vi "CL-3000 sample.vi"() -> ()   [LabVIEW 2020]
uses:
  ctrl/select_out.ctl
  ctrl/select_group.ctl
  Public/enums/CL3IF_PEAKNO.ctl
  Public/clusters/CL3IF_ETHERNET_SETTING.ctl
  Public/enums/CL3IF_SELECTED_INDEX.ctl
  Public/enums/CL3IF_OUTNO.ctl
  Public/enums/CL3IF_ZERO_GROUP.ctl
  Keyence CL-3000.lvlib
panel:
  out "pulase_reset":bool=TRUE
  out "mask_left_1":bool
  in  "display point num":u16=2 min=2 max=10000
  out "data num":u16
  out "mask_right":bool
  out "No Wave":string="\nNo Wave"
  out "log1":dbl[][](graph)
  out "log2":dbl[][](graph)
  out "log3":dbl[][](graph)
  out "log4":dbl[][](graph)
  out "log5":dbl[][](graph)
  out "log6":dbl[][](graph)
  out "log7":dbl[][](graph)
  out "select_out_last":T1
  out "log8":dbl[][](graph)
  in  "timeout":u32=5000 caption="Timeout"
  in  "path":path
  out "mask_left_2":bool
  in  "on_off_group":bool
  out "Result_8":string caption="Result"
  out "Result_4":string caption="Result"
  out "Result_7":string caption="Result"
  in  "select_group":T2
  out "Result_5":string caption="Result"
  out "Result_6":string caption="Result"
  in  "light_ctrl_off":bool
  in  "light_ctrl_on":bool
  in  "meas_ctrl_off":bool
  in  "meas_ctrl_on":bool
  out "Result_2":string caption="Result"
  in  "peak4":bool
  in  "peak3":bool
  in  "peak2":bool
  in  "peak1":bool
  out "Light Graph":dbl[][](graph)
  in  "selectedIndex":enum16{"OLDEST", "NEWEST"}(ring)
  in  "request_data":u32=10000 caption="Request\nData" min=1 max=10000
  in  "save_csv_file":bool
  in  "select_out_graph":T1
  in  "select_out_command":T1
  in  "on_off":bool
  in  "reset_pulse_count":bool
  out "pulse_count":i32 caption="Pulse Count"
  in  "get_pulse_count":bool
  out "program_no":u8 caption="Get Program No"
  in  "get_program_no":bool
  in  "switch_program_no":u8 caption="Switch Program No" max=7
  in  "switch_program":bool
  out "Result_3":string caption="Result"
  in  "reset_group":bool
  in  "reset_multi":bool
  in  "timing_group":bool
  in  "timing_multi":bool
  in  "auto_zero_group":bool
  in  "auto_zero_multi":bool
  out "Result_1":string caption="Result"
  in  "IP Address":u8[](array[numeric])=[192, 168, 1, 1]
  in  "Comm Interface":enum8{"USB", "ETHERNET"}(ring)
  in  "LabVIEW stop":bool
  in  "clear_storage_data":bool
  in  "stop_storage":bool
  in  "start_storage":bool
  out "storage_index":u32 caption="Index"
  out "Measurement Data":T3(array[cluster])=[{"Out No"=1, "Value"=0, "valueInfo"=enum."VALID", "judgeResult"=0}, {"Out No"=2, "Value"=0, "valueInfo"=enum."VALID", "judgeResult"=0}, {"Out No"=3, "Value"=0, "valueInfo"=enum."VALID", "judgeResult"=0}, {"Out No"=4, "Value"=0, "valueInfo"=enum."VALID", "judgeResult"=0}, {"Out No"=5, "Value"=0, "valueInfo"=enum."VALID", "judgeResult"=0}, {"Out No"=6, "Value"=0, "valueInfo"=enum."VALID", "judgeResult"=0}, {"Out No"=7, "Value"=0, "valueInfo"=enum."VALID", "judgeResult"=0}, {"Out No"=8, "Value"=0, "valueInfo"=enum."VALID", "judgeResult"=0}] {"judgeResult" items=["HI"=1, "GO"=2, "LO"=4, "**"=5, "--"=0]}
  in  "get_light_stop":bool
  in  "get_trend_stop":bool
  in  "close":bool
  in  "Port":u32
  in  "Head":u8 max=5
  in  "get_light_start":bool
  in  "select_graph":enum8{"TriggerCount", "PulseCount"}(ring)
  in  "get_storage_data":bool
  in  "get_storage_index":bool
  in  "get_trend_start":bool
  out "trend_index":u32 caption="Index"
  in  "get_trend_index":bool
  in  "open":bool
  in  "Device ID":i32 min=0 max=2
  out "Trend Graph":T4(graph)
  # "Judgement\nResult"
  # "Measurement Data"
  # "ValueInfo"
  # "Out No"
  # "Value"
  # "ver 1.0.0"
  # "Trend DATA"
  # "Storage DATA"
  # "Light"
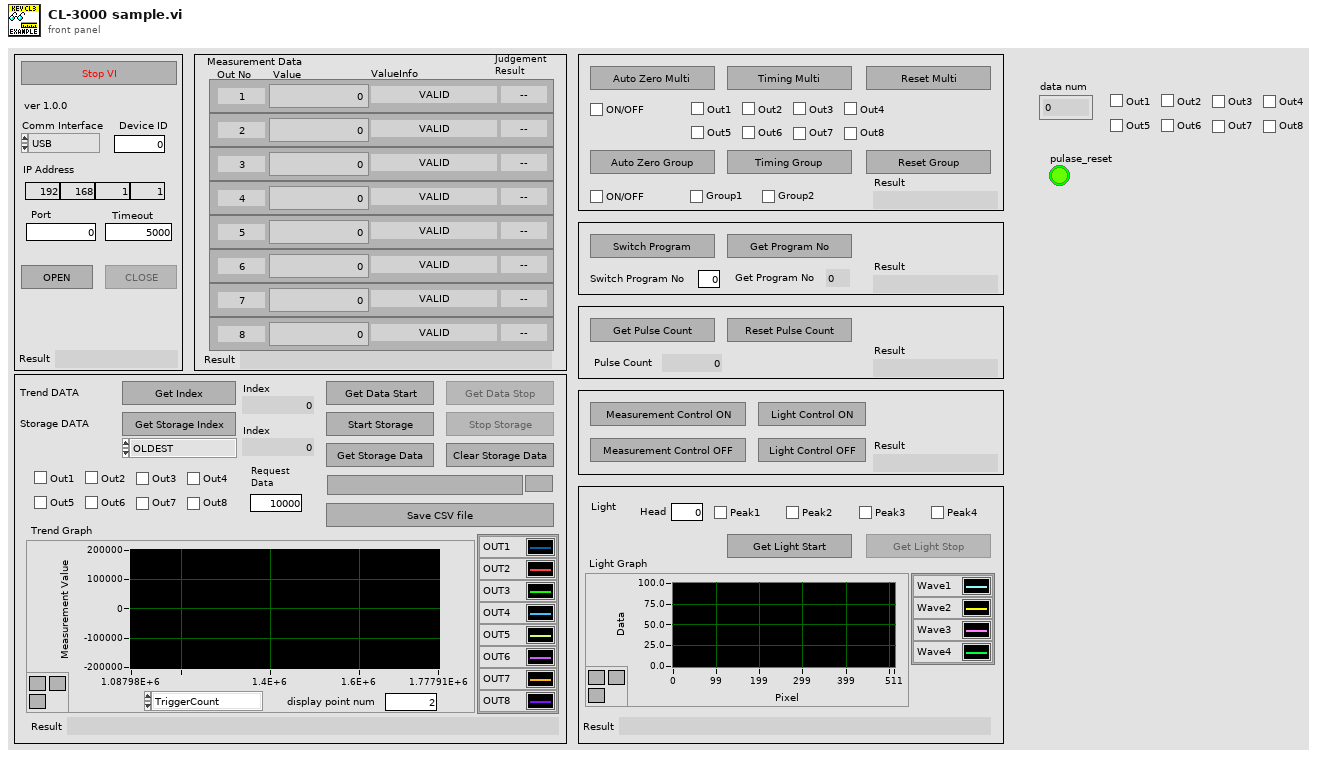
[diagram p1: front panel]
types:
  T1 = typedef "select_out.ctl" = cluster{"out1":bool, "out2":bool, "out3":bool, "out4":bool, "out5":bool, "out6":bool, "out7":bool, "out8":bool}
  T2 = typedef "select_group.ctl" = cluster{"group1":bool, "group2":bool}
  T3 = cluster{"Out No":i32, "Value":i32, "valueInfo":enum8{"VALID", "JUDGMENTSTANDBY", "INVALID", "OVERDISPRANGE_P", "OVERDISPRANGE_N"}, "judgeResult":u16}[]
  T4 = cluster{cluster{"triggerCount":dbl, "measurementValue":dbl}[]}[]
  T5 = enum8{"Enabled", "Disabled", "Disabled and Grayed Out"}
  T6 = cluster{cluster{"triggerCount":u32, "measurementValue":i32}[]}[]
  T7 = typedef "Keyence CL-3000.lvlib/CL3IF_ETHERNET_SETTING.ctl" = cluster{"IP Address":cluster{"IP1":u8, "IP2":u8, "IP3":u8, "IP4":u8}, "portNo":u32}
  T8 = cluster{cluster{"triggerCount":u32, "measurementValue":dbl}[]}[]
  T9 = typedef "Keyence CL-3000.lvlib/CL3IF_SELECTED_INDEX.ctl" = enum16{"OLDEST", "NEWEST"}
  T10 = typedef "Keyence CL-3000.lvlib/CL3IF_MEASUREMENT_DATA.ctl" = cluster{"addInfo":cluster{"triggerCount":u32, "pulseCount":i32}, "outMeasurementData":T11[]}
  T11 = typedef "Keyence CL-3000.lvlib/CL3IF_OUTMEASUREMENT_DATA.ctl" = cluster{"measurementValue":i32, "valueInfo":T12, "judgeResult":T13}
  T12 = typedef "Keyence CL-3000.lvlib/CL3IF_VALUE_INFO.ctl" = enum8{"VALID", "JUDGMENTSTANDBY", "INVALID", "OVERDISPRANGE_P", "OVERDISPRANGE_N"}
  T13 = typedef "Keyence CL-3000.lvlib/CL3IF_JUDGE_RESULT.ctl" = u8
  T14 = cluster{i32, "measurementValue":i32, "valueInfo":T12, "judgeResult":T13}
  T15 = cluster{cluster{"Count":dbl, "measurementValue":dbl}[]}[]
  T16 = typedef "Keyence CL-3000.lvlib/CL3IF_PEAKNO.ctl" = u16
  T17 = cluster{"IP Address":u8, "IP Address":u8, "IP Address":u8, "IP Address":u8}
  T18 = typedef "Keyence CL-3000.lvlib/CL3IF_OUTNO.ctl" = u16
  T19 = typedef "Keyence CL-3000.lvlib/CL3IF_ZERO_GROUP.ctl" = u16
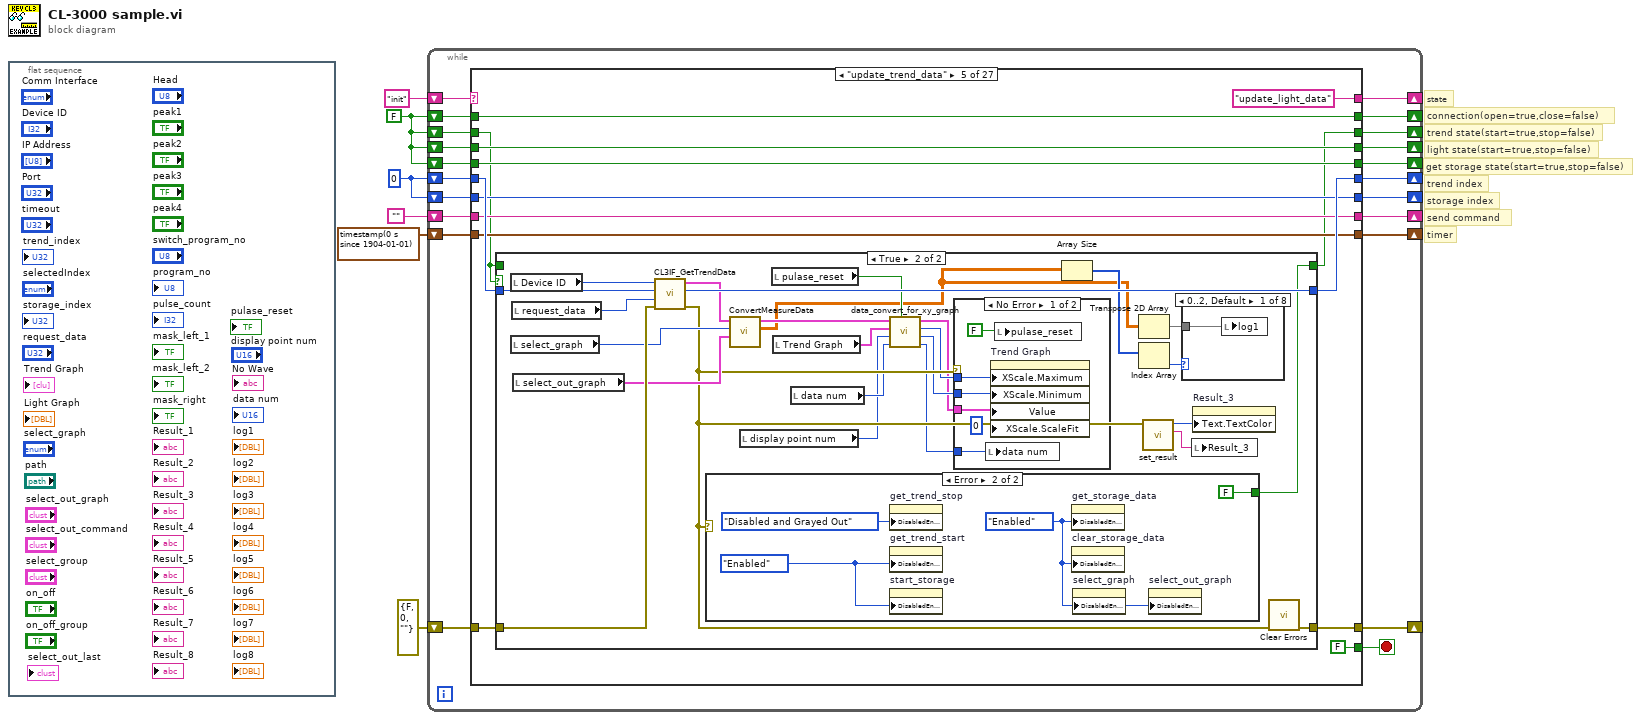
[diagram p0: block diagram]
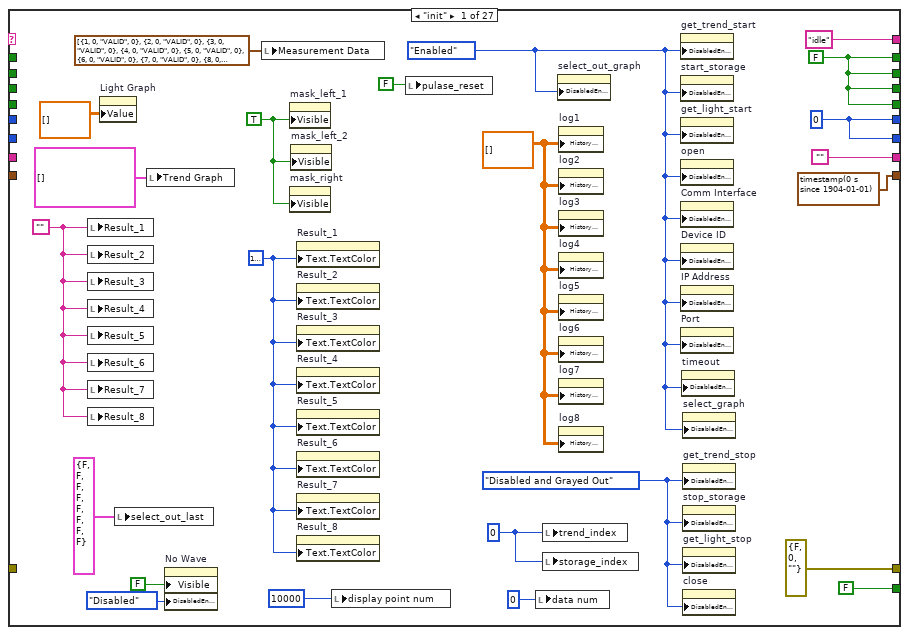
[diagram p2: hidden frame]
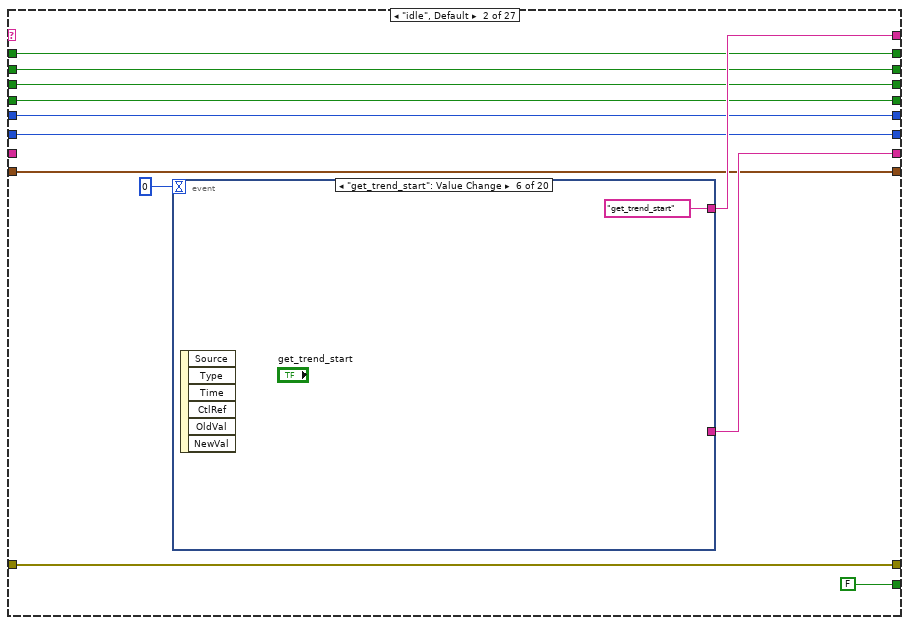
[diagram p3: hidden frame]
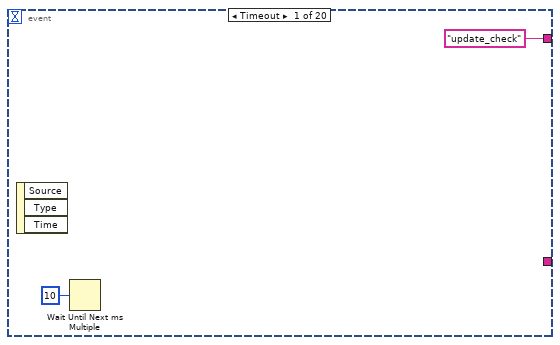
[diagram p4: hidden frame]
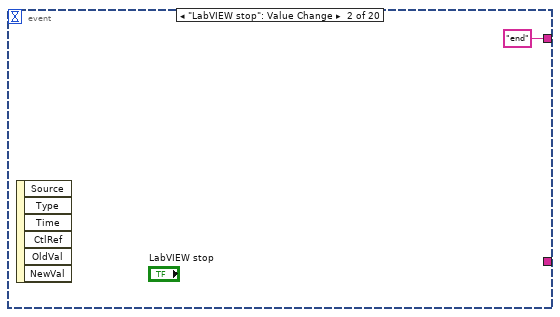
[diagram p5: hidden frame]
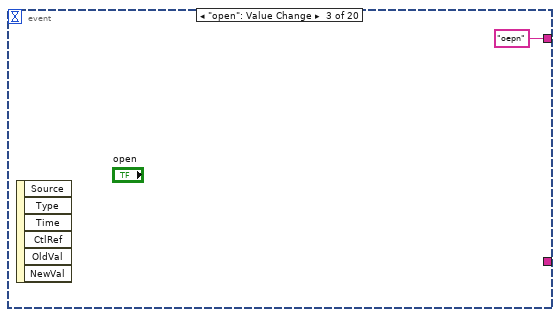
[diagram p6: hidden frame]
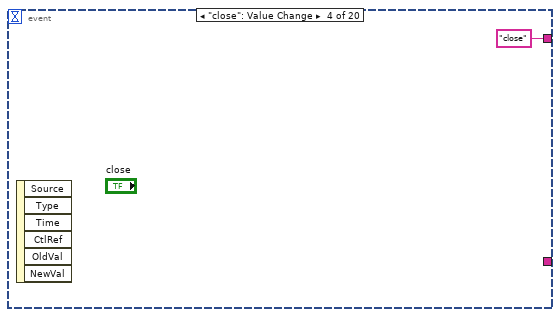
[diagram p7: hidden frame]
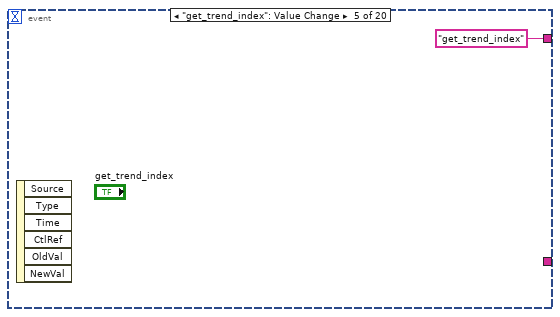
[diagram p8: hidden frame]
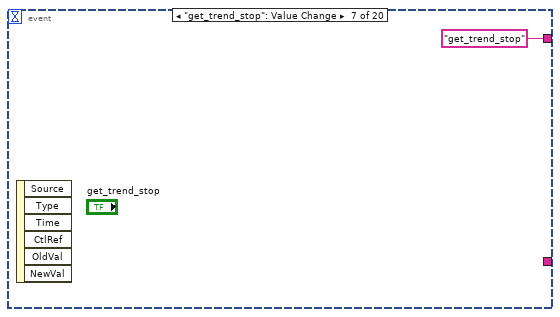
[diagram p9: hidden frame]
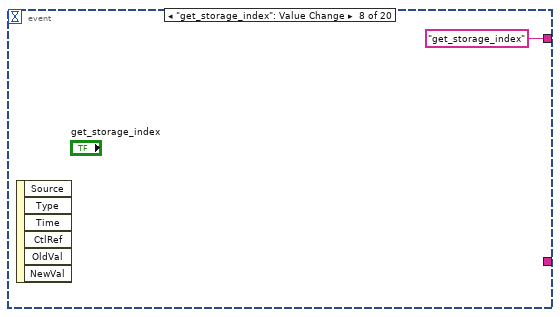
[diagram p10: hidden frame]
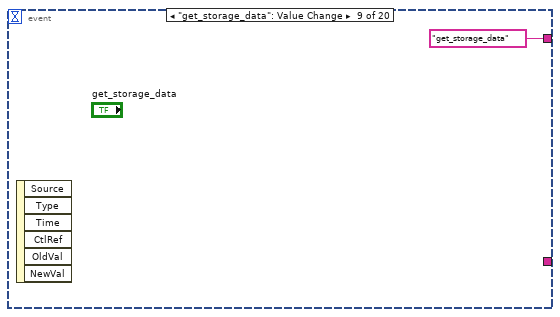
[diagram p11: hidden frame]
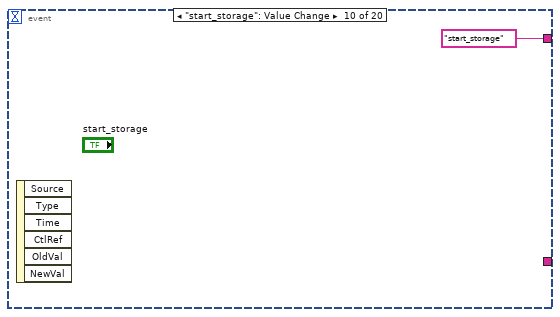
[diagram p12: hidden frame]
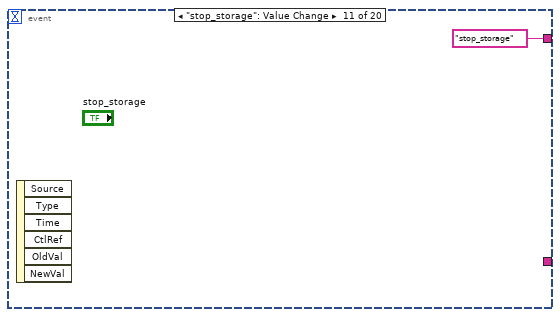
[diagram p13: hidden frame]
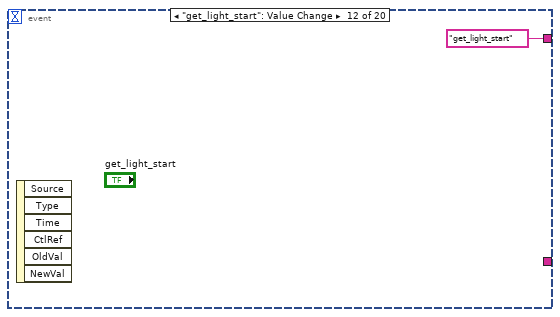
[diagram p14: hidden frame]
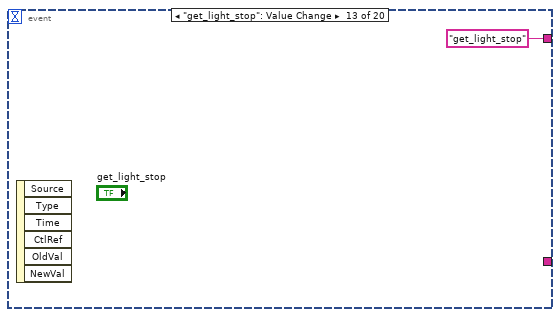
[diagram p15: hidden frame]
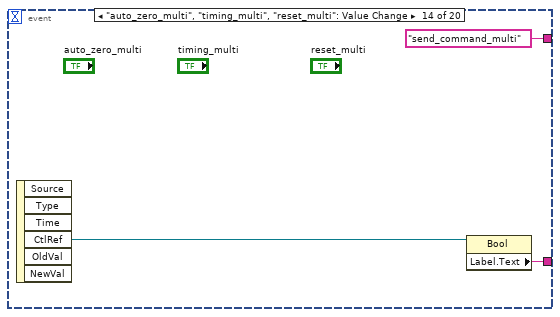
[diagram p16: hidden frame]
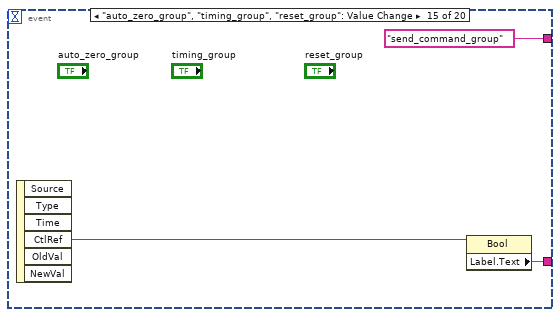
[diagram p17: hidden frame]
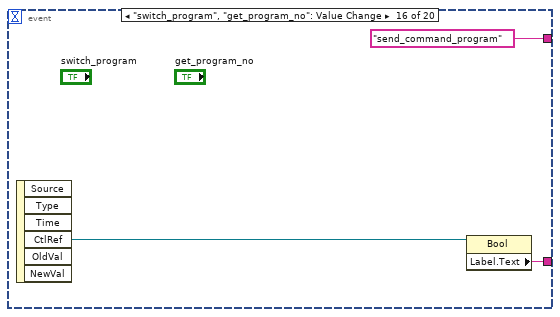
[diagram p18: hidden frame]
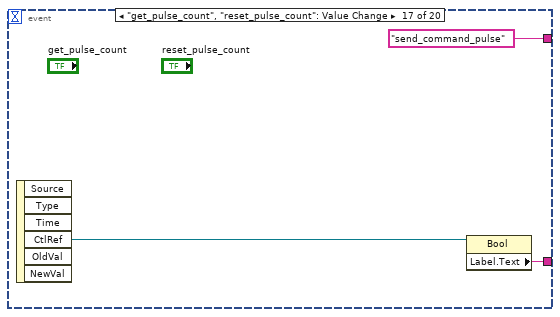
[diagram p19: hidden frame]
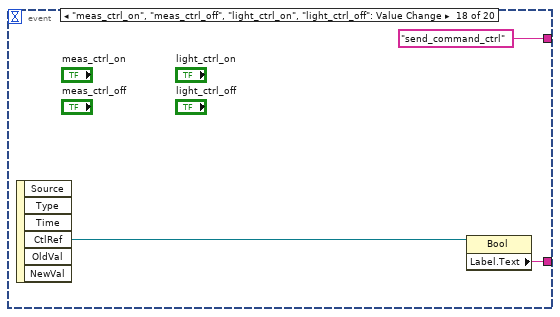
[diagram p20: hidden frame]
diagram:
  w5 = u32 0 ("Index")
  w3 = FALSE
  # "get storage state(start=true,stop=false)"
  # "timer"
  # "send command"
  # "light state(start=true,stop=false)"
  # "storage index"
  # "trend index"
  # "trend state(start=true,stop=false)"
  # "connection(open=true,close=false)"
  # "state"
  n1 = flat-sequence {
    frame #0 {
    }
  }
  n2 = while {
    shift-right: [w26] -> _
    shift-left: "init" -> [w27]
    shift-right: [w25] -> _
    shift-left: errorcluster {"status"=FALSE, "code"=0, "source"=""} ("error") -> [w24]
    shift-right: [w21] -> _
    shift-left: w3 -> [w22]
    shift-right: [w19] -> _
    shift-left: w3 -> [w20]
    shift-right: [w18] -> _
    shift-left: w5 -> [w17]
    shift-right: [w16] -> _
    shift-left: w5 -> [w15]
    shift-right: [w13] -> _
    shift-left: w3 -> [w14]
    shift-right: [w12] -> _
    shift-left: "" ("Result") -> [w11]
    shift-right: [w10] -> _
    shift-left: timestamp(0 s since 1904-01-01) -> [w9]
    shift-right: [w7] -> _
    shift-left: w3 -> [w8]
    stop <- w23 stop-if-true
    n3 = case shown="\"update_trend_data\"" w27 {
      tunnel: ["idle" w59 w103 "update_trend_data" "update_light_data" "update_storage_data" "error" "error" "error" "error" "error" "error" "error" "error" "error" "error" "error" "error" "error" "error" "error" "error" "error" "error" "error" "idle" "end"] -> w26
      tunnel: [errorcluster {"status"=FALSE, "code"=0, "source"=""} ("error") w62 w107 w116 w148 w215 w268 w325 w366 w377 w391 w421 w440 w453 w460 w476 w506 w522 w543 w600 w643 w678 w704 w736 w758 w800 errorcluster {"status"=FALSE, "code"=0, "source"=""} ("error")] -> w25
      tunnel: w24 -> [_ w62 w107 w123 w154 w216 w269 w346 w362 w386 w397 w421 w440 w453 w468 w483 w512 w529 w573 w612 w646 w681 w707 w739 w757 w801 w810]
      tunnel: [FALSE FALSE FALSE FALSE FALSE FALSE FALSE FALSE FALSE FALSE FALSE FALSE FALSE FALSE FALSE FALSE FALSE FALSE FALSE FALSE FALSE FALSE FALSE FALSE FALSE FALSE TRUE] -> w23
      tunnel: w22 -> [_ w58 w113 w124 w155 w217 w270 _ _ w387 w402 w428 w441 w454 w471 w489 w517 w534 w578 w617 w648 w686 w712 w744 w766 w799 _]
      tunnel: [w38 w58 w113 w124 w155 w217 w270 w338 w358 w387 w402 w428 w441 w454 w471 w489 w517 w534 w578 w617 w648 w686 w712 w744 w766 w799 w814] -> w21
      tunnel: w20 -> [_ w57 w111 w121 w145 w214 w267 w336 _ w383 _ w426 _ w448 w470 w488 w515 w532 w575 w614 w636 w683 w709 w741 w763 w798 _]
      tunnel: [w38 w57 w111 w121 w144 w214 w267 w336 w358 w383 TRUE w426 FALSE w448 w470 w488 w515 w532 w575 w614 w636 w683 w709 w741 w763 w798 w814] -> w19
      tunnel: [w46 w56 w112 w122 w152 w212 w266 w337 w371 w382 w396 w424 w437 w452 w469 w487 w514 w531 w577 w616 w637 w685 w711 w743 w765 w797 w817] -> w18
      tunnel: w17 -> [_ w56 w112 w122 w153 w212 w266 w337 w371 w382 _ w424 w437 w452 w469 w487 w514 w531 w577 w616 w638 w685 w711 w743 w765 w797 _]
      tunnel: [w46 w55 w110 w120 w151 w213 w260 w335 w370 w381 w400 w427 w436 w451 w465 w477 w513 w530 w576 w615 w635 w684 w710 w742 w764 w796 w817] -> w16
      tunnel: w15 -> [_ w55 w110 w120 w151 w213 w261 w335 w370 w381 w400 w427 w436 w451 w465 _ w513 w530 w576 w615 w635 w684 w710 w742 w764 w796 _]
      tunnel: w14 -> [_ w54 w109 w119 w150 w208 w265 w334 _ w380 w399 _ w435 _ w464 w486 w516 w533 w574 w613 w647 w682 w708 w740 _ w795 _]
      tunnel: [w38 w54 w109 w119 w150 w207 w265 w334 w358 w380 w399 TRUE w435 FALSE w464 w486 w516 w533 w574 w613 w647 w682 w708 w740 FALSE w795 w814] -> w13
      tunnel: ["" w53 w108 w118 w149 w211 w264 w327 w369 w379 w395 w420 w434 w446 w462 w485 w510 w527 w540 w597 w640 w675 w701 w735 w761 w794 ""] -> w12
      tunnel: w11 -> [_ _ w108 w118 w149 w211 w264 w327 w369 w379 w395 w420 w434 w446 w462 w485 w510 w527 w540 w597 w640 w675 w701 w735 w761 w794 _]
      tunnel: [timestamp(0 s since 1904-01-01) w52 w98 w117 w147 w210 w263 w326 w367 w378 w394 w419 w433 w445 w461 w484 w509 w526 w544 w601 w644 w679 w705 w737 w760 w793 timestamp(0 s since 1904-01-01)] -> w10
      tunnel: w9 -> [_ w52 w100 w117 w147 w210 w263 w326 w367 w378 w394 w419 w433 w445 w461 w484 w509 w526 w544 w601 w644 w679 w705 w737 w760 w793 _]
      tunnel: w8 -> [_ w51 w97 w115 w146 w209 w262 w322 _ w374 w390 w418 w432 w444 w457 _ w505 w523 w539 w596 w639 w674 w700 w732 w759 w792 _]
      tunnel: [w38 w51 w97 w115 w146 w209 w259 w322 w358 w374 w390 w418 w432 w444 w457 w475 w505 w523 w539 w596 w639 w674 w700 w732 w759 w792 w814] -> w7
      frame "init" {
        w30 = u32 0 ("trend_index")
        w34 = dbl[][] []
        w41 = u32 16777228
        w45 = TRUE
        w37 = T5."Disabled and Grayed Out"
        w36 = T5."Enabled"
        w46 = u32 0 ("Index")
        w38 = FALSE
        w42 = "" ("Result")
        n4 = local write "Result_1"(w42) -> ()
        n5 = local write "Result_2"(w42) -> ()
        n6 = local write "Result_3"(w42) -> ()
        n7 = local write "Result_4"(w42) -> ()
        n8 = local write "Result_5"(w42) -> ()
        n9 = local write "Result_6"(w42) -> ()
        n10 = local write "Result_7"(w42) -> ()
        n11 = local write "Result_8"(w42) -> ()
        n12 = property on="Light Graph" class="WFGraph (strict)"("Value"=dbl[][] [] ("Light Graph")) -> ()  [unwired: 2 in, 2 out]
        n13 = local write "select_out_last"(T1 {"out1"=FALSE, "out2"=FALSE, "out3"=FALSE, "out4"=FALSE, "out5"=FALSE, "out6"=FALSE, "out7"=FALSE, "out8"=FALSE} ("select_out_last")) -> ()
        n14 = local write "Trend Graph"(T6 [] ("Trend Graph")) -> ()
        n15 = property on="No Wave" class="Str"("Visible"=FALSE, "DisabledEnum"=T5."Disabled") -> ()  [unwired: 2 in, 2 out]
        n16 = local write "Measurement Data"(T3 [{"Out No"=1, "Value"=0, "valueInfo"=enum."VALID", "judgeResult"=0}, {"Out No"=2, "Value"=0, "valueInfo"=enum."VALID", "judgeResult"=0}, {"Out No"=3, "Value"=0, "valueInfo"=enum."VALID", "judgeResult"=0}, {"Out No"=4, "Value"=0, "valueInfo"=enum."VALID", "judgeResult"=0}, {"Out No"=5, "Value"=0, "valueInfo"=enum."VALID", "judgeResult"=0}, {"Out No"=6, "Value"=0, "valueInfo"=enum."VALID", "judgeResult"=0}, {"Out No"=7, "Value"=0, "valueInfo"=enum."VALID", "judgeResult"=0}, {"Out No"=8, "Value"=0, "valueInfo"=enum."VALID", "judgeResult"=0}] ("Measurement Data")) -> ()
        n17 = property on="mask_left_1" class="Bool (strict)"("Visible"=w45) -> ()  [unwired: 2 in, 2 out]
        n18 = property on="mask_right" class="Bool (strict)"("Visible"=w45) -> ()  [unwired: 2 in, 2 out]
        n19 = property on="mask_left_2" class="Bool (strict)"("Visible"=w45) -> ()  [unwired: 2 in, 2 out]
        n20 = property on="Result_1" class="Str"("Text.TextColor"=w41) -> ()  [unwired: 2 in, 2 out]
        n21 = property on="Result_2" class="Str"("Text.TextColor"=w41) -> ()  [unwired: 2 in, 2 out]
        n22 = property on="Result_3" class="Str"("Text.TextColor"=w41) -> ()  [unwired: 2 in, 2 out]
        n23 = property on="Result_4" class="Str"("Text.TextColor"=w41) -> ()  [unwired: 2 in, 2 out]
        n24 = property on="Result_5" class="Str"("Text.TextColor"=w41) -> ()  [unwired: 2 in, 2 out]
        n25 = property on="Result_6" class="Str"("Text.TextColor"=w41) -> ()  [unwired: 2 in, 2 out]
        n26 = property on="Result_7" class="Str"("Text.TextColor"=w41) -> ()  [unwired: 2 in, 2 out]
        n27 = property on="Result_8" class="Str"("Text.TextColor"=w41) -> ()  [unwired: 2 in, 2 out]
        n28 = local write "display point num"(u16 10000 ("disp num")) -> ()
        n29 = local write "pulase_reset"(FALSE) -> ()
        n30 = local write "data num"(u16 0 ("data num in")) -> ()
        n31 = local write "trend_index"(w30) -> ()
        n32 = local write "storage_index"(w30) -> ()
        n33 = property on="select_out_graph" class="Clust (strict)"("DisabledEnum"=w36) -> ()  [unwired: 2 in, 2 out]
        n34 = property on="log1" class="WFChart (strict)"("History Data"=w34) -> ()  [unwired: 2 in, 2 out]
        n35 = property on="log2" class="WFChart (strict)"("History Data"=w34) -> ()  [unwired: 2 in, 2 out]
        n36 = property on="log3" class="WFChart (strict)"("History Data"=w34) -> ()  [unwired: 2 in, 2 out]
        n37 = property on="log4" class="WFChart (strict)"("History Data"=w34) -> ()  [unwired: 2 in, 2 out]
        n38 = property on="log5" class="WFChart (strict)"("History Data"=w34) -> ()  [unwired: 2 in, 2 out]
        n39 = property on="log6" class="WFChart (strict)"("History Data"=w34) -> ()  [unwired: 2 in, 2 out]
        n40 = property on="log7" class="WFChart (strict)"("History Data"=w34) -> ()  [unwired: 2 in, 2 out]
        n41 = property on="log8" class="WFChart (strict)"("History Data"=w34) -> ()  [unwired: 2 in, 2 out]
        n42 = property on="get_trend_start" class="Bool"("DisabledEnum"=w36) -> ()  [unwired: 2 in, 2 out]
        n43 = property on="start_storage" class="Bool"("DisabledEnum"=w36) -> ()  [unwired: 2 in, 2 out]
        n44 = property on="get_light_start" class="Bool"("DisabledEnum"=w36) -> ()  [unwired: 2 in, 2 out]
        n45 = property on="open" class="Bool"("DisabledEnum"=w36) -> ()  [unwired: 2 in, 2 out]
        n46 = property on="Comm Interface" class="Enum (strict)"("DisabledEnum"=w36) -> ()  [unwired: 2 in, 2 out]
        n47 = property on="Device ID" class="DigNum (strict)"("DisabledEnum"=w36) -> ()  [unwired: 2 in, 2 out]
        n48 = property on="IP Address" class="Arr (strict)"("DisabledEnum"=w36) -> ()  [unwired: 2 in, 2 out]
        n49 = property on="Port" class="DigNum (strict)"("DisabledEnum"=w36) -> ()  [unwired: 2 in, 2 out]
        n50 = property on="timeout" class="DigNum (strict)"("DisabledEnum"=w36) -> ()  [unwired: 2 in, 2 out]
        n51 = property on="select_graph" class="Enum (strict)"("DisabledEnum"=w36) -> ()  [unwired: 2 in, 2 out]
        n52 = property on="get_trend_stop" class="Bool"("DisabledEnum"=w37) -> ()  [unwired: 2 in, 2 out]
        n53 = property on="stop_storage" class="Bool"("DisabledEnum"=w37) -> ()  [unwired: 2 in, 2 out]
        n54 = property on="get_light_stop" class="Bool"("DisabledEnum"=w37) -> ()  [unwired: 2 in, 2 out]
        n55 = property on="close" class="Bool"("DisabledEnum"=w37) -> ()  [unwired: 2 in, 2 out]
      }
      frame "idle", Default {
        n56 = event shown="[5] \"get_trend_start\": Value Change" {
          selector: _ -> [_ _ _ _ _ _ _ _ _ _ _ _ _ _ _ _ _ _ _ _]
          dyn-events: _ -> [_ _ _ _ _ _ _ _ _ _ _ _ _ _ _ _ _ _ _ _]
          timeout: 0 -> [_ _ _ _ _ _ _ _ _ _ _ _ _ _ _ _ _ _ _ _]
          tunnel: ["update_check" "end" "oepn" "close" "get_trend_index" "get_trend_start" "get_trend_stop" "get_storage_index" "get_storage_data" "start_storage" "stop_storage" "get_light_start" "get_light_stop" "send_command_multi" "send_command_group" "send_command_program" "send_command_pulse" "send_command_ctrl" "send_command_clear_storage" "save_csv_file"] -> w59
          tunnel: [_ _ _ _ _ _ _ _ _ _ _ _ _ w77 w80 w83 w86 w89 w93 _] -> w53
          event Timeout {
            n57 = event-data() -> ()  [unwired: 1 in, 3 out]
            n58 = Wait Until Next ms Multiple(millisecond multiple=u32 10) -> ()  [unwired: 1 out]
          }
          event "LabVIEW stop": Value Change {
            n59 = event-data() -> ()  [unwired: 1 in, 6 out]
          }
          event "open": Value Change {
            n60 = event-data() -> ()  [unwired: 1 in, 6 out]
          }
          event "close": Value Change {
            n61 = event-data() -> ()  [unwired: 1 in, 6 out]
          }
          event "get_trend_index": Value Change {
            n62 = event-data() -> ()  [unwired: 1 in, 6 out]
          }
          event "get_trend_start": Value Change {
            n63 = event-data() -> ()  [unwired: 1 in, 6 out]
          }
          event "get_trend_stop": Value Change {
            n64 = event-data() -> ()  [unwired: 1 in, 6 out]
          }
          event "get_storage_index": Value Change {
            n65 = event-data() -> ()  [unwired: 1 in, 6 out]
          }
          event "get_storage_data": Value Change {
            n66 = event-data() -> ()  [unwired: 1 in, 6 out]
          }
          event "start_storage": Value Change {
            n67 = event-data() -> ()  [unwired: 1 in, 6 out]
          }
          event "stop_storage": Value Change {
            n68 = event-data() -> ()  [unwired: 1 in, 6 out]
          }
          event "get_light_start": Value Change {
            n69 = event-data() -> ()  [unwired: 1 in, 6 out]
          }
          event "get_light_stop": Value Change {
            n70 = event-data() -> ()  [unwired: 1 in, 6 out]
          }
          event "auto_zero_multi", "timing_multi", "reset_multi": Value Change {
            n71 = event-data() -> ("CtlRef"=w78:refnum<vi>)  [unwired: 1 in, 5 out]
            n72 = property class="Bool"(reference=w78) -> ("Label.Text"=w77:string)  [unwired: 1 in, 2 out]
          }
          event "auto_zero_group", "timing_group", "reset_group": Value Change {
            n73 = event-data() -> ("CtlRef"=w81:refnum<vi>)  [unwired: 1 in, 5 out]
            n74 = property class="Bool"(reference=w81) -> ("Label.Text"=w80:string)  [unwired: 1 in, 2 out]
          }
          event "switch_program", "get_program_no": Value Change {
            n75 = event-data() -> ("CtlRef"=w84:refnum<vi>)  [unwired: 1 in, 5 out]
            n76 = property class="Bool"(reference=w84) -> ("Label.Text"=w83:string)  [unwired: 1 in, 2 out]
          }
          event "get_pulse_count", "reset_pulse_count": Value Change {
            n77 = event-data() -> ("CtlRef"=w87:refnum<vi>)  [unwired: 1 in, 5 out]
            n78 = property class="Bool"(reference=w87) -> ("Label.Text"=w86:string)  [unwired: 1 in, 2 out]
          }
          event "meas_ctrl_on", "meas_ctrl_off", "light_ctrl_on", "light_ctrl_off": Value Change {
            n79 = event-data() -> ("CtlRef"=w90:refnum<vi>)  [unwired: 1 in, 5 out]
            n80 = property class="Bool"(reference=w90) -> ("Label.Text"=w89:string)  [unwired: 1 in, 2 out]
          }
          event "clear_storage_data": Value Change {
            n81 = event-data() -> ("CtlRef"=w94:refnum<vi>)  [unwired: 1 in, 5 out]
            n82 = local write "Result_3"("") -> ()
            n83 = property class="Bool"(reference=w94) -> ("Label.Text"=w93:string)  [unwired: 1 in, 2 out]
          }
          event "save_csv_file": Value Change {
            n84 = event-data() -> ()  [unwired: 1 in, 6 out]
          }
        }
      }
      frame "update_check" {
        n85 = Get Date/Time In Seconds() -> (seconds since 1Jan1904=w99:timestamp)
        n86 = Add(x=w100, y=0.1) -> (x+y=w105:timestamp)
        n87 = Greater?(x=w99, y=w105) -> (0:w101:bool)
        n88 = Select(t=w99, s=w101, f=w100) -> (s? t:f=w98:timestamp)
        n89 = Select(t="update_measurement_data", s=w101, f="error") -> (s? t:f=w103:string)
      }
      frame "update_measurement_data" {
        n90 = case shown="True" w124 {
          tunnel: w123 -> [w127 w135]
          tunnel: [w127 w128] -> w116
          frame False {
          }
          frame True {
            n91 = local read "Device ID"() -> (w136:i32)
            n92 = call "CL3IF_GetMeasurementData.vi"("error in"=w135, "deviceId"=w136) -> ("error out"=w129:errorcluster, "MEASUREMENT_DATA"=w134:T10)  [unwired: 8 in]
            n93 = Unbundle By Name(w134) -> ("outMeasurementData"=w133:T11[])
            n94 = for {
              tunnel: w133 -> [w143] mode=indexing
              tunnel: [w142] -> w132 mode=indexing
              i -> [w141]
              n95 = Unbundle By Name(w143) -> ("measurementValue"=w139:i32, "valueInfo"=w138:T12, "judgeResult"=w137:T13)
              n96 = Increment(x=w141) -> (x+1=w140:i32)
              n97 = Bundle(w140, "measurementValue"=w139, "valueInfo"=w138, "judgeResult"=w137) -> (w142:T14)  [unwired: 1 in]
            }
            "Measurement Data" <- w132
            n98 = call "set_result.vi"("error in"=w129) -> ("string"=w130:string, "font color"=w131:u32)  [unwired: 9 in]
            n99 = local write "Result_2"(w130) -> ()
            n100 = property on="Result_2" class="Str"("Text.TextColor"=w131) -> ()  [unwired: 2 in, 2 out]
            n101 = call <vilib>:"Clear Errors.vi"("error in (no error)"=w129) -> ("error out"=w128:errorcluster)  [unwired: 5 in, 1 out]
          }
        }
      }
      frame "update_trend_data" {
        n102 = case shown="True" w145 {
          tunnel: w154 -> [w160 w179]
          tunnel: [w160 w176] -> w148
          tunnel: w153 -> [w159 w180]
          tunnel: [w159 w186] -> w152
          tunnel: w145 -> [w158 _]
          tunnel: [w158 w170] -> w144
          frame False {
          }
          frame True {
            n103 = local read "Device ID"() -> (w181:i32)
            n104 = local read "select_graph"() -> (w175:enum8{"TriggerCount", "PulseCount"})
            n105 = local read "request_data"() -> (w185:u32)
            n106 = local read "select_out_graph"() -> (w174:T1)
            n107 = call "CL3IF_GetTrendData.vi"("error in"=w179, "requestDataCount"=w185, "index"=w180, "deviceId"=w181) -> ("error out"=w169:errorcluster, "nextIndex"=w186:u32, "measurementData"=w184:T10[])  [unwired: 3 in, 2 out]
            n108 = case shown="Error" w169 {
              tunnel: [TRUE FALSE] -> w170
              frame No Error {
              }
              frame Error {
                w204 = T5."Enabled"
                w206 = T5."Enabled"
                n109 = property on="get_trend_stop" class="Bool"("DisabledEnum"=T5."Disabled and Grayed Out") -> ()  [unwired: 2 in, 2 out]
                n110 = property on="get_trend_start" class="Bool"("DisabledEnum"=w206) -> ()  [unwired: 2 in, 2 out]
                n111 = property on="start_storage" class="Bool"("DisabledEnum"=w206) -> ()  [unwired: 2 in, 2 out]
                n112 = property on="get_storage_data" class="Bool"("DisabledEnum"=w204) -> ()  [unwired: 2 in, 2 out]
                n113 = property on="clear_storage_data" class="Bool"("DisabledEnum"=w204) -> ()  [unwired: 2 in, 2 out]
                n114 = property on="select_graph" class="Enum (strict)"("DisabledEnum"=w204) -> ()  [unwired: 2 in, 2 out]
                n115 = property on="select_out_graph" class="Clust (strict)"("DisabledEnum"=w204) -> ()  [unwired: 2 in, 2 out]
              }
            }
            n116 = call "ConvertMeasureData.vi"("select_out_graph"=w174, "select_graph"=w175, "measurementData"=w184) -> ("Log out"=w161:dbl[][], "Data out"=w182:T15)  [unwired: 7 in]
            n117 = local read "display point num"() -> (w163:u16)
            n118 = local read "pulase_reset"() -> (w162:bool)
            n119 = local read "Trend Graph"() -> (w183:T4)
            n120 = local read "data num"() -> (w166:u16)
            n121 = call "data_convert_for_xy_graph.vi"("pulse reset"=w162, "data num in"=w166, "disp num"=w163, "graph data in"=w183, "new data in"=w182) -> ("data num out"=w165:u16, "min"=w167:i64, "max"=w168:i64, "data out"=w164:T15)  [unwired: 3 in]
            n122 = case shown="No Error" w169 {
              tunnel: w168 -> [w191 _]
              tunnel: w167 -> [w190 _]
              tunnel: w165 -> [w192 _]
              tunnel: w164 -> [w189 _]
              frame No Error {
                n123 = local write "data num"(w192) -> ()
                n124 = property on="Trend Graph" class="XYGraph (strict)"("XScale.Maximum"=w191, "XScale.Minimum"=w190, "Value"=w189, "XScale.ScaleFit"=u8 0 ("Xスケール.スケールフィット")) -> ()  [unwired: 2 in, 2 out]
                n125 = local write "pulase_reset"(FALSE ("ブール")) -> ()
              }
              frame Error {
                n126 = local write "pulase_reset"(FALSE ("ブール")) -> ()
              }
            }
            n127 = Array Size(array=w161) -> (size(s)=w173:i32[])
            n128 = Transpose 2D Array(2D array=w161) -> (transposed array=w171:dbl[][])
            n129 = Index Array(array=w173) -> (element=w172:i32)  [unwired: 1 in]
            n130 = call "set_result.vi"("error in"=w169) -> ("string"=w178:string, "font color"=w177:u32)  [unwired: 9 in]
            n131 = case shown="0..2, Default" w172 {
              tunnel: w171 -> [w194 w195 w196 w197 w198 w199 w200 w201]
              frame 0..2, Default {
                n132 = local write "log1"(w194) -> ()
              }
              frame 3 {
                n133 = local write "log2"(w195) -> ()
              }
              frame 4 {
                n134 = local write "log3"(w196) -> ()
              }
              frame 5 {
                n135 = local write "log4"(w197) -> ()
              }
              frame 6 {
                n136 = local write "log5"(w198) -> ()
              }
              frame 7 {
                n137 = local write "log6"(w199) -> ()
              }
              frame 8 {
                n138 = local write "log7"(w200) -> ()
              }
              frame 9 {
                n139 = local write "log8"(w201) -> ()
              }
            }
            n140 = local write "Result_3"(w178) -> ()
            n141 = property on="Result_3" class="Str"("Text.TextColor"=w177) -> ()  [unwired: 2 in, 2 out]
            n142 = call <vilib>:"Clear Errors.vi"("error in (no error)"=w169) -> ("error out"=w176:errorcluster)  [unwired: 5 in, 1 out]
          }
        }
      }
      frame "update_light_data" {
        n143 = case shown="True" w208 {
          tunnel: w216 -> [w221 w228]
          tunnel: [w221 w222] -> w215
          tunnel: w208 -> [w220 _]
          tunnel: [w220 w223] -> w207
          frame False {
          }
          frame True {
            w233 = T16 8 items=["CL3IF_PEAKNO_01"=1, "CL3IF_PEAKNO_02"=2, "CL3IF_PEAKNO_03"=4, "CL3IF_PEAKNO_04"=8] ("peakNo")
            w234 = T16 4 items=["CL3IF_PEAKNO_01"=1, "CL3IF_PEAKNO_02"=2, "CL3IF_PEAKNO_03"=4, "CL3IF_PEAKNO_04"=8] ("peakNo")
            w235 = T16 2 items=["CL3IF_PEAKNO_01"=1, "CL3IF_PEAKNO_02"=2, "CL3IF_PEAKNO_03"=4, "CL3IF_PEAKNO_04"=8] ("peakNo")
            w240 = T16 1 items=["CL3IF_PEAKNO_01"=1, "CL3IF_PEAKNO_02"=2, "CL3IF_PEAKNO_03"=4, "CL3IF_PEAKNO_04"=8] ("peakNo")
            w236 = T16 0 items=["CL3IF_PEAKNO_01"=1, "CL3IF_PEAKNO_02"=2, "CL3IF_PEAKNO_03"=4, "CL3IF_PEAKNO_04"=8] ("peakNo")
            n144 = local read "Head"() -> (w245:u8)
            n145 = local read "peak1"() -> (w241:bool)
            n146 = local read "peak2"() -> (w239:bool)
            n147 = local read "peak3"() -> (w238:bool)
            n148 = local read "peak4"() -> (w237:bool)
            n149 = local read "Device ID"() -> (w246:i32)
            n150 = Select(t=w240, s=w241, f=w236) -> (s? t:f=w232:T16)
            n151 = Select(t=w235, s=w239, f=w236) -> (s? t:f=w231:T16)
            n152 = Select(t=w234, s=w238, f=w236) -> (s? t:f=w230:T16)
            n153 = Select(t=w233, s=w237, f=w236) -> (s? t:f=w229:T16)
            n154 = Compound Arithmetic op=OR(w232, w231, w230, w229) -> (w243:T16)
            n155 = call "CL3IF_GetLightWaveform.vi"("error in"=w228, "peakNo"=w243, "headNo"=w245, "deviceId"=w246) -> ("error out"=w224:errorcluster, "waveData"=w244:u16[])  [unwired: 6 in]
            n156 = for {
              N: 4 -> [_]
              tunnel: w244 -> [w254]
              tunnel: [w255] -> w225 mode=indexing
              i -> [w258]
              w256 = 512
              n157 = Multiply(x=w256, y=w258) -> (x*y=w257:i32)
              n158 = Array Subset(array=w254, index=w257, length=w256) -> (w255:u16[])
            }
            n159 = case shown="Error" w224 {
              tunnel: w224 -> [_ w250]
              tunnel: [TRUE FALSE] -> w223
              frame No Error {
              }
              frame Error {
                n160 = Unbundle By Name(w250) -> ("code"=w249:i32)
                n161 = case shown="81055" w249 {
                  frame Default {
                  }
                  frame 528469 {
                    n162 = property on="No Wave" class="Str"("Visible"=TRUE) -> ()  [unwired: 2 in, 2 out]
                  }
                }
                n163 = property on="get_light_start" class="Bool"("DisabledEnum"=T5."Enabled") -> ()  [unwired: 2 in, 2 out]
                n164 = property on="get_light_stop" class="Bool"("DisabledEnum"=T5."Disabled and Grayed Out") -> ()  [unwired: 2 in, 2 out]
              }
            }
            n165 = local write "Light Graph"(w225) -> ()
            n166 = call "set_result.vi"("error in"=w224) -> ("string"=w226:string, "font color"=w227:u32)  [unwired: 9 in]
            n167 = local write "Result_8"(w226) -> ()
            n168 = property on="Result_8" class="Str"("Text.TextColor"=w227) -> ()  [unwired: 2 in, 2 out]
            n169 = call <vilib>:"Clear Errors.vi"("error in (no error)"=w224) -> ("error out"=w222:errorcluster)  [unwired: 5 in, 1 out]
          }
        }
      }
      frame "update_storage_data" {
        n170 = case shown="True" w262 {
          selector: w262 -> [w273 w284]
          tunnel: w269 -> [w275 w287]
          tunnel: [w275 w282] -> w268
          tunnel: w261 -> [w274 w289]
          tunnel: [w274 w288] -> w260
          tunnel: [w273 w283] -> w259
          frame False {
          }
          frame True {
            n171 = local read "Device ID"() -> (w286:i32)
            n172 = local read "request_data"() -> (w285:u32)
            n173 = call "CL3IF_GetStorageData.vi"("error in"=w287, "requestDataCount"=w285, "index"=w289, "deviceId"=w286) -> ("error out"=w277:errorcluster, "nextIndex"=w288:u32, "measurementData"=w281:T10[])  [unwired: 3 in, 2 out]
            n174 = case shown="No Error" w277 {
              tunnel: w284 -> [w310 _]
              tunnel: [w310 FALSE] -> w283
              tunnel: w281 -> [w307 _]
              frame No Error {
                n175 = local read "select_graph"() -> (w306:enum8{"TriggerCount", "PulseCount"})
                n176 = local read "select_out_graph"() -> (w305:T1)
                n177 = local read "display point num"() -> (w296:u16)
                n178 = local read "Trend Graph"() -> (w309:T4)
                n179 = local read "data num"() -> (w298:u16)
                n180 = call "ConvertMeasureData.vi"("select_out_graph"=w305, "select_graph"=w306, "measurementData"=w307) -> ("Log out"=w303:dbl[][], "Data out"=w308:T15)  [unwired: 7 in]
                n181 = Array Size(array=w303) -> (size(s)=w302:i32[])
                n182 = Transpose 2D Array(2D array=w303) -> (transposed array=w304:dbl[][])
                n183 = call "data_convert_for_xy_graph.vi"("pulse reset"=FALSE, "data num in"=w298, "disp num"=w296, "graph data in"=w309, "new data in"=w308) -> ("data num out"=w297:u16, "min"=w300:i64, "max"=w299:i64, "data out"=w295:T15)  [unwired: 3 in]
                n184 = Index Array(array=w302) -> (element=w301:i32)  [unwired: 1 in]
                n185 = case shown="0..2, Default" w301 {
                  tunnel: w304 -> [w311 w312 w313 w314 w315 w316 w317 w318]
                  frame 0..2, Default {
                    n186 = local write "log1"(w311) -> ()
                  }
                  frame 3 {
                    n187 = local write "log2"(w312) -> ()
                  }
                  frame 4 {
                    n188 = local write "log3"(w313) -> ()
                  }
                  frame 5 {
                    n189 = local write "log4"(w314) -> ()
                  }
                  frame 6 {
                    n190 = local write "log5"(w315) -> ()
                  }
                  frame 7 {
                    n191 = local write "log6"(w316) -> ()
                  }
                  frame 8 {
                    n192 = local write "log7"(w317) -> ()
                  }
                  frame 9 {
                    n193 = local write "log8"(w318) -> ()
                  }
                }
                n194 = property on="Trend Graph" class="XYGraph (strict)"("XScale.Maximum"=w299, "XScale.Minimum"=w300, "Value"=w295, "XScale.ScaleFit"=u8 0 ("Xスケール.スケールフィット")) -> ()  [unwired: 2 in, 2 out]
                n195 = local write "data num"(w297) -> ()
              }
              frame Error {
                w319 = T5."Enabled"
                n196 = property on="select_out_graph" class="Clust (strict)"("DisabledEnum"=w319) -> ()  [unwired: 2 in, 2 out]
                n197 = property on="get_trend_start" class="Bool"("DisabledEnum"=w319) -> ()  [unwired: 2 in, 2 out]
                n198 = property on="start_storage" class="Bool"("DisabledEnum"=w319) -> ()  [unwired: 2 in, 2 out]
                n199 = property on="clear_storage_data" class="Bool"("DisabledEnum"=w319) -> ()  [unwired: 2 in, 2 out]
                n200 = property on="get_storage_data" class="Bool"("DisabledEnum"=w319) -> ()  [unwired: 2 in, 2 out]
                n201 = property on="select_graph" class="Enum (strict)"("DisabledEnum"=w319) -> ()  [unwired: 2 in, 2 out]
              }
            }
            n202 = Unbundle By Name(w277) -> ("code"=w276:i32)
            n203 = case shown="81055" w276 {
              tunnel: w277 -> [w290 w292]
              tunnel: [w290 w291] -> w278
              frame 0, Default {
              }
              frame 528469 {
                n204 = call <vilib>:"Clear Errors.vi"("error in (no error)"=w292) -> ("error out"=w291:errorcluster)  [unwired: 5 in, 1 out]
              }
            }
            n205 = call "set_result.vi"("error in"=w278) -> ("string"=w279:string, "font color"=w280:u32)  [unwired: 9 in]
            n206 = local write "Result_3"(w279) -> ()
            n207 = property on="Result_3" class="Str"("Text.TextColor"=w280) -> ()  [unwired: 2 in, 2 out]
            n208 = call <vilib>:"Clear Errors.vi"("error in (no error)"=w278) -> ("error out"=w282:errorcluster)  [unwired: 5 in, 1 out]
          }
        }
      }
      frame "oepn" {
        w343 = T5."Disabled and Grayed Out"
        w344 = T5."Enabled"
        n209 = local read "IP Address"() -> (w333:u8[])
        n210 = local read "Port"() -> (w339:u32)
        n211 = Index Array(array=w333) -> (element #1=w331:u8, element #2=w332:u8, element #3=w330:u8, element #4=w329:u8)  [unwired: 4 in]
        n212 = local read "Comm Interface"() -> (w341:enum8{"USB", "ETHERNET"})
        n213 = local read "Device ID"() -> (w340:i32)
        n214 = local read "timeout"() -> (w321:u32)
        n215 = Bundle("IP Address"=w331, "IP Address"=w332, "IP Address"=w330, "IP Address"=w329) -> (w328:T17)  [unwired: 1 in]
        n216 = Bundle By Name(cluster=T7 {"IP Address"={"IP1"=0, "IP2"=0, "IP3"=0, "IP4"=0}, "portNo"=0} ("ethernetSetting"), "IP Address"=w328, "portNo"=w339) -> (w347:T7)
        n217 = call "Initialize.vi"("Comm Interface"=w341, "error in (no error)"=w346, "ethernetSetting"=w347, "timeout"=w321, "deviceId"=w340) -> ("error out"=w325:errorcluster)  [unwired: 6 in]
        n218 = case shown="No Error" w325 {
          tunnel: [TRUE FALSE] -> w338
          frame No Error {
            w352 = FALSE
            w351 = T5."Disabled and Grayed Out"
            n219 = property on="mask_right" class="Bool (strict)"("Visible"=w352) -> ()  [unwired: 2 in, 2 out]
            n220 = property on="mask_left_1" class="Bool (strict)"("Visible"=w352) -> ()  [unwired: 2 in, 2 out]
            n221 = property on="mask_left_2" class="Bool (strict)"("Visible"=w352) -> ()  [unwired: 2 in, 2 out]
            n222 = property on="Comm Interface" class="Enum (strict)"("DisabledEnum"=w351) -> ()  [unwired: 2 in, 2 out]
            n223 = property on="Device ID" class="DigNum (strict)"("DisabledEnum"=w351) -> ()  [unwired: 2 in, 2 out]
            n224 = property on="IP Address" class="Arr (strict)"("DisabledEnum"=w351) -> ()  [unwired: 2 in, 2 out]
            n225 = property on="Port" class="DigNum (strict)"("DisabledEnum"=w351) -> ()  [unwired: 2 in, 2 out]
            n226 = property on="timeout" class="DigNum (strict)"("DisabledEnum"=w351) -> ()  [unwired: 2 in, 2 out]
          }
          frame Error {
          }
        }
        n227 = Select(t=w344, s=w325, f=w343) -> (s? t:f=w345:T5)
        n228 = Select(t=w343, s=w325, f=w344) -> (s? t:f=w342:T5)
        n229 = property on="open" class="Bool"("DisabledEnum"=w345) -> ()  [unwired: 2 in, 2 out]
        n230 = property on="close" class="Bool"("DisabledEnum"=w342) -> ()  [unwired: 2 in, 2 out]
        n231 = call "set_result.vi"("error in"=w325) -> ("string"=w323:string, "font color"=w324:u32)  [unwired: 9 in]
        n232 = property on="Result_1" class="Str"("Text.TextColor"=w324) -> ()  [unwired: 2 in, 2 out]
        n233 = local write "Result_1"(w323) -> ()
      }
      frame "close" {
        w356 = T5."Enabled"
        w368 = TRUE
        w358 = FALSE
        w359 = T5."Disabled and Grayed Out"
        w363 = T5."Enabled"
        n234 = local read "Device ID"() -> (w360:i32)
        n235 = property on="mask_left_1" class="Bool (strict)"("Visible"=w368) -> ()  [unwired: 2 in, 2 out]
        n236 = property on="No Wave" class="Str"("Visible"=FALSE) -> ()  [unwired: 2 in, 2 out]
        n237 = property on="mask_right" class="Bool (strict)"("Visible"=w368) -> ()  [unwired: 2 in, 2 out]
        n238 = property on="mask_left_2" class="Bool (strict)"("Visible"=w368) -> ()  [unwired: 2 in, 2 out]
        n239 = call "CL3IF_StopStorage.vi"("error in"=w362, "deviceId"=w360) -> ("error out"=w357:errorcluster)  [unwired: 9 in]
        n240 = call <vilib>:"Clear Errors.vi"("error in (no error)"=w357) -> ("error out"=w361:errorcluster)  [unwired: 5 in, 1 out]
        n241 = call "Close.vi"("error in (no error)"=w361, "deviceId"=w360) -> ("error out"=w366:errorcluster)  [unwired: 9 in]
        n242 = property on="open" class="Bool"("DisabledEnum"=w363) -> ()  [unwired: 2 in, 2 out]
        n243 = property on="Comm Interface" class="Enum (strict)"("DisabledEnum"=w363) -> ()  [unwired: 2 in, 2 out]
        n244 = property on="Device ID" class="DigNum (strict)"("DisabledEnum"=w363) -> ()  [unwired: 2 in, 2 out]
        n245 = property on="IP Address" class="Arr (strict)"("DisabledEnum"=w363) -> ()  [unwired: 2 in, 2 out]
        n246 = property on="Port" class="DigNum (strict)"("DisabledEnum"=w363) -> ()  [unwired: 2 in, 2 out]
        n247 = property on="timeout" class="DigNum (strict)"("DisabledEnum"=w363) -> ()  [unwired: 2 in, 2 out]
        n248 = call "set_result.vi"("error in"=w366) -> ("string"=w364:string, "font color"=w365:u32)  [unwired: 9 in]
        n249 = local write "Result_1"(w364) -> ()
        n250 = property on="Result_1" class="Str"("Text.TextColor"=w365) -> ()  [unwired: 2 in, 2 out]
        n251 = property on="get_trend_start" class="Bool"("DisabledEnum"=w356) -> ()  [unwired: 2 in, 2 out]
        n252 = property on="start_storage" class="Bool"("DisabledEnum"=w356) -> ()  [unwired: 2 in, 2 out]
        n253 = property on="get_storage_data" class="Bool"("DisabledEnum"=w356) -> ()  [unwired: 2 in, 2 out]
        n254 = property on="clear_storage_data" class="Bool"("DisabledEnum"=w356) -> ()  [unwired: 2 in, 2 out]
        n255 = property on="get_light_start" class="Bool"("DisabledEnum"=w356) -> ()  [unwired: 2 in, 2 out]
        n256 = property on="select_graph" class="Enum (strict)"("DisabledEnum"=w356) -> ()  [unwired: 2 in, 2 out]
        n257 = property on="select_out_graph" class="Clust (strict)"("DisabledEnum"=w356) -> ()  [unwired: 2 in, 2 out]
        n258 = property on="close" class="Bool"("DisabledEnum"=w359) -> ()  [unwired: 2 in, 2 out]
        n259 = property on="stop_storage" class="Bool"("DisabledEnum"=w359) -> ()  [unwired: 2 in, 2 out]
        n260 = property on="get_trend_stop" class="Bool"("DisabledEnum"=w359) -> ()  [unwired: 2 in, 2 out]
        n261 = property on="get_light_stop" class="Bool"("DisabledEnum"=w359) -> ()  [unwired: 2 in, 2 out]
      }
      frame "get_trend_index" {
        n262 = local read "Device ID"() -> (w385:i32)
        n263 = call "CL3IF_GetTrendIndex.vi"("error in"=w386, "deviceId"=w385) -> ("error out"=w377:errorcluster, "index"=w384:u32)  [unwired: 8 in]
        n264 = local write "trend_index"(w384) -> ()
        n265 = call "set_result.vi"("error in"=w377) -> ("string"=w376:string, "font color"=w375:u32)  [unwired: 9 in]
        n266 = local write "Result_3"(w376) -> ()
        n267 = property on="Result_3" class="Str"("Text.TextColor"=w375) -> ()  [unwired: 2 in, 2 out]
      }
      frame "get_trend_start" {
        # "1"
        n268 = local read "Device ID"() -> (w398:i32)
        n269 = call "CL3IF_GetTrendIndex.vi"("error in"=w397, "deviceId"=w398) -> ("error out"=w391:errorcluster, "index"=w396:u32)  [unwired: 8 in]
        n270 = case shown="No Error" w391 {
          frame No Error {
            w406 = 0.0
            w410 = dbl[][] []
            w411 = T5."Disabled and Grayed Out"
            n271 = local read "select_graph"() -> (w413:enum8{"TriggerCount", "PulseCount"})
            n272 = case shown="\"PulseCount\"" w413 {
              tunnel: ["Trigger" "Pulse"] -> w412
              frame "TriggerCount", Default {
              }
              frame "PulseCount" {
              }
            }
            n273 = property on="get_trend_stop" class="Bool"("DisabledEnum"=T5."Enabled") -> ()  [unwired: 2 in, 2 out]
            n274 = local write "data num"(u16 0 ("data num in")) -> ()
            n275 = local write "Trend Graph"(T8 [{array[10000 elements]}, {array[10000 elements]}, {array[10000 elements]}, {array[10000 elements]}, {array[10000 elements]}, {array[10000 elements]}, {array[10000 elements]}, {array[10000 elements]}]) -> ()
            n276 = local read "select_out_graph"() -> (w409:T1)
            n277 = property on="Trend Graph" class="XYGraph (strict)"("XScale.Minimum"=w406, "XScale.Maximum"=w406, "XScale.NameLbl.Text"=w412, "XScale.ScaleFit"=u8 0) -> ()  [unwired: 2 in, 2 out]
            n278 = property on="get_trend_start" class="Bool"("DisabledEnum"=w411) -> ()  [unwired: 2 in, 2 out]
            n279 = property on="start_storage" class="Bool"("DisabledEnum"=w411) -> ()  [unwired: 2 in, 2 out]
            n280 = property on="get_storage_data" class="Bool"("DisabledEnum"=w411) -> ()  [unwired: 2 in, 2 out]
            n281 = property on="clear_storage_data" class="Bool"("DisabledEnum"=w411) -> ()  [unwired: 2 in, 2 out]
            n282 = property on="select_graph" class="Enum (strict)"("DisabledEnum"=w411) -> ()  [unwired: 2 in, 2 out]
            n283 = local write "select_out_last"(w409) -> ()
            n284 = property on="select_out_graph" class="Clust (strict)"("DisabledEnum"=w411) -> ()  [unwired: 2 in, 2 out]
            n285 = property on="log1" class="WFChart (strict)"("History Data"=w410) -> ()  [unwired: 2 in, 2 out]
            n286 = property on="log2" class="WFChart (strict)"("History Data"=w410) -> ()  [unwired: 2 in, 2 out]
            n287 = property on="log3" class="WFChart (strict)"("History Data"=w410) -> ()  [unwired: 2 in, 2 out]
            n288 = property on="log4" class="WFChart (strict)"("History Data"=w410) -> ()  [unwired: 2 in, 2 out]
            n289 = property on="log5" class="WFChart (strict)"("History Data"=w410) -> ()  [unwired: 2 in, 2 out]
            n290 = property on="log6" class="WFChart (strict)"("History Data"=w410) -> ()  [unwired: 2 in, 2 out]
            n291 = property on="log7" class="WFChart (strict)"("History Data"=w410) -> ()  [unwired: 2 in, 2 out]
            n292 = property on="log8" class="WFChart (strict)"("History Data"=w410) -> ()  [unwired: 2 in, 2 out]
          }
          frame Error {
          }
        }
        n293 = call "set_result.vi"("error in"=w391) -> ("string"=w393:string, "font color"=w392:u32)  [unwired: 9 in]
        n294 = local write "Result_3"(w393) -> ()
        n295 = property on="Result_3" class="Str"("Text.TextColor"=w392) -> ()  [unwired: 2 in, 2 out]
      }
      frame "get_light_start" {
        n296 = property on="get_light_start" class="Bool"("DisabledEnum"=T5."Disabled and Grayed Out") -> ()  [unwired: 2 in, 2 out]
        n297 = property on="get_light_stop" class="Bool"("DisabledEnum"=T5."Enabled") -> ()  [unwired: 2 in, 2 out]
        n298 = property on="No Wave" class="Str"("Visible"=FALSE) -> ()  [unwired: 2 in, 2 out]
      }
      frame "get_trend_stop" {
        w431 = T5."Enabled"
        n299 = property on="get_trend_stop" class="Bool"("DisabledEnum"=T5."Disabled and Grayed Out") -> ()  [unwired: 2 in, 2 out]
        n300 = property on="get_trend_start" class="Bool"("DisabledEnum"=w431) -> ()  [unwired: 2 in, 2 out]
        n301 = property on="start_storage" class="Bool"("DisabledEnum"=w431) -> ()  [unwired: 2 in, 2 out]
        n302 = property on="get_storage_data" class="Bool"("DisabledEnum"=w431) -> ()  [unwired: 2 in, 2 out]
        n303 = property on="clear_storage_data" class="Bool"("DisabledEnum"=w431) -> ()  [unwired: 2 in, 2 out]
        n304 = property on="select_graph" class="Enum (strict)"("DisabledEnum"=w431) -> ()  [unwired: 2 in, 2 out]
        n305 = property on="select_out_graph" class="Clust (strict)"("DisabledEnum"=w431) -> ()  [unwired: 2 in, 2 out]
      }
      frame "get_light_stop" {
        n306 = property on="get_light_start" class="Bool"("DisabledEnum"=T5."Enabled") -> ()  [unwired: 2 in, 2 out]
        n307 = property on="get_light_stop" class="Bool"("DisabledEnum"=T5."Disabled and Grayed Out") -> ()  [unwired: 2 in, 2 out]
      }
      frame "get_storage_index" {
        n308 = local read "selectedIndex"() -> (w463:enum16{"OLDEST", "NEWEST"})
        n309 = local read "Device ID"() -> (w466:i32)
        n310 = call "CL3IF_GetStorageIndex.vi"("error in"=w468, "selectedIndex"=w463, "deviceId"=w466) -> ("error out"=w460:errorcluster, "index"=w467:u32)  [unwired: 7 in]
        n311 = local write "storage_index"(w467) -> ()
        n312 = call "set_result.vi"("error in"=w460) -> ("string"=w458:string, "font color"=w459:u32)  [unwired: 9 in]
        n313 = local write "Result_3"(w458) -> ()
        n314 = property on="Result_3" class="Str"("Text.TextColor"=w459) -> ()  [unwired: 2 in, 2 out]
      }
      frame "get_storage_data" {
        n315 = local read "Device ID"() -> (w478:i32)
        n316 = call "CL3IF_GetStorageIndex.vi"("error in"=w483, "selectedIndex"=CL3IF_SELECTED_INDEX."OLDEST", "deviceId"=w478) -> ("error out"=w479:errorcluster, "index"=w477:u32)  [unwired: 7 in]
        n317 = call "CL3IF_GetStorageData.vi"("error in"=w479, "requestDataCount"=u32 1, "index"=w477, "deviceId"=w478) -> ("error out"=w476:errorcluster)  [unwired: 3 in, 4 out]
        n318 = case shown="No Error" w476 {
          tunnel: [TRUE FALSE] -> w475
          frame No Error {
            w494 = dbl[][] []
            w499 = T5."Disabled and Grayed Out" ("無効")
            w501 = 0.0
            n319 = local read "select_graph"() -> (w493:enum8{"TriggerCount", "PulseCount"})
            n320 = property on="log1" class="WFChart (strict)"("History Data"=w494) -> ()  [unwired: 2 in, 2 out]
            n321 = property on="log2" class="WFChart (strict)"("History Data"=w494) -> ()  [unwired: 2 in, 2 out]
            n322 = property on="log3" class="WFChart (strict)"("History Data"=w494) -> ()  [unwired: 2 in, 2 out]
            n323 = property on="log4" class="WFChart (strict)"("History Data"=w494) -> ()  [unwired: 2 in, 2 out]
            n324 = case shown="\"TriggerCount\", Default" w493 {
              tunnel: ["Trigger" "Pulse"] -> w492
              frame "TriggerCount", Default {
              }
              frame "PulseCount" {
              }
            }
            n325 = property on="log5" class="WFChart (strict)"("History Data"=w494) -> ()  [unwired: 2 in, 2 out]
            n326 = property on="log6" class="WFChart (strict)"("History Data"=w494) -> ()  [unwired: 2 in, 2 out]
            n327 = property on="log7" class="WFChart (strict)"("History Data"=w494) -> ()  [unwired: 2 in, 2 out]
            n328 = property on="log8" class="WFChart (strict)"("History Data"=w494) -> ()  [unwired: 2 in, 2 out]
            n329 = local write "data num"(u16 0 ("data num in")) -> ()
            n330 = local read "select_out_graph"() -> (w498:T1)
            n331 = property on="get_trend_start" class="Bool"("DisabledEnum"=w499) -> ()  [unwired: 2 in, 2 out]
            n332 = property on="start_storage" class="Bool"("DisabledEnum"=w499) -> ()  [unwired: 2 in, 2 out]
            n333 = property on="clear_storage_data" class="Bool"("DisabledEnum"=w499) -> ()  [unwired: 2 in, 2 out]
            n334 = property on="get_storage_data" class="Bool"("DisabledEnum"=w499) -> ()  [unwired: 2 in, 2 out]
            n335 = property on="select_graph" class="Enum (strict)"("DisabledEnum"=w499) -> ()  [unwired: 2 in, 2 out]
            n336 = property on="Trend Graph" class="XYGraph (strict)"("XScale.Minimum"=w501, "XScale.Maximum"=w501, "XScale.ScaleFit"=u8 0, "XScale.NameLbl.Text"=w492) -> ()  [unwired: 2 in, 2 out]
            n337 = local write "Trend Graph"(T8 [{array[10000 elements]}, {array[10000 elements]}, {array[10000 elements]}, {array[10000 elements]}, {array[10000 elements]}, {array[10000 elements]}, {array[10000 elements]}, {array[10000 elements]}]) -> ()
            n338 = local write "select_out_last"(w498) -> ()
            n339 = property on="select_out_graph" class="Clust (strict)"("DisabledEnum"=w499) -> ()  [unwired: 2 in, 2 out]
          }
          frame Error {
          }
        }
        n340 = call "set_result.vi"("error in"=w476) -> ("string"=w480:string, "font color"=w481:u32)  [unwired: 9 in]
        n341 = local write "Result_3"(w480) -> ()
        n342 = property on="Result_3" class="Str"("Text.TextColor"=w481) -> ()  [unwired: 2 in, 2 out]
      }
      frame "start_storage" {
        n343 = local read "Device ID"() -> (w511:i32)
        n344 = call "CL3IF_StartStorage.vi"("error in"=w512, "deviceId"=w511) -> ("error out"=w506:errorcluster)  [unwired: 9 in]
        n345 = case shown="No Error" w506 {
          frame No Error {
            w520 = T5."Disabled and Grayed Out"
            n346 = property on="get_trend_start" class="Bool"("DisabledEnum"=w520) -> ()  [unwired: 2 in, 2 out]
            n347 = property on="start_storage" class="Bool"("DisabledEnum"=w520) -> ()  [unwired: 2 in, 2 out]
            n348 = property on="get_storage_data" class="Bool"("DisabledEnum"=w520) -> ()  [unwired: 2 in, 2 out]
            n349 = property on="clear_storage_data" class="Bool"("DisabledEnum"=w520) -> ()  [unwired: 2 in, 2 out]
            n350 = property on="stop_storage" class="Bool"("DisabledEnum"=T5."Enabled") -> ()  [unwired: 2 in, 2 out]
          }
          frame Error {
          }
        }
        n351 = call "set_result.vi"("error in"=w506) -> ("string"=w507:string, "font color"=w508:u32)  [unwired: 9 in]
        n352 = local write "Result_3"(w507) -> ()
        n353 = property on="Result_3" class="Str"("Text.TextColor"=w508) -> ()  [unwired: 2 in, 2 out]
      }
      frame "stop_storage" {
        n354 = local read "Device ID"() -> (w528:i32)
        n355 = call "CL3IF_StopStorage.vi"("error in"=w529, "deviceId"=w528) -> ("error out"=w522:errorcluster)  [unwired: 9 in]
        n356 = case shown="No Error" w522 {
          frame No Error {
            w537 = T5."Enabled"
            n357 = property on="get_trend_start" class="Bool"("DisabledEnum"=w537) -> ()  [unwired: 2 in, 2 out]
            n358 = property on="start_storage" class="Bool"("DisabledEnum"=w537) -> ()  [unwired: 2 in, 2 out]
            n359 = property on="get_storage_data" class="Bool"("DisabledEnum"=w537) -> ()  [unwired: 2 in, 2 out]
            n360 = property on="clear_storage_data" class="Bool"("DisabledEnum"=w537) -> ()  [unwired: 2 in, 2 out]
            n361 = property on="stop_storage" class="Bool"("DisabledEnum"=T5."Disabled and Grayed Out") -> ()  [unwired: 2 in, 2 out]
          }
          frame Error {
          }
        }
        n362 = call "set_result.vi"("error in"=w522) -> ("string"=w524:string, "font color"=w525:u32)  [unwired: 9 in]
        n363 = local write "Result_3"(w524) -> ()
        n364 = property on="Result_3" class="Str"("Text.TextColor"=w525) -> ()  [unwired: 2 in, 2 out]
      }
      frame "send_command_multi" {
        w554 = T18 128 items=["OUT01"=1, "OUT02"=2, "OUT03"=4, "OUT04"=8, "OUT05"=16, "OUT06"=32, "OUT07"=64, "OUT08"=128, "ALL OUT"=255] ("outNo")
        w555 = T18 64 items=["OUT01"=1, "OUT02"=2, "OUT03"=4, "OUT04"=8, "OUT05"=16, "OUT06"=32, "OUT07"=64, "OUT08"=128, "ALL OUT"=255] ("outNo")
        w556 = T18 32 items=["OUT01"=1, "OUT02"=2, "OUT03"=4, "OUT04"=8, "OUT05"=16, "OUT06"=32, "OUT07"=64, "OUT08"=128, "ALL OUT"=255] ("outNo")
        w557 = T18 16 items=["OUT01"=1, "OUT02"=2, "OUT03"=4, "OUT04"=8, "OUT05"=16, "OUT06"=32, "OUT07"=64, "OUT08"=128, "ALL OUT"=255] ("outNo")
        w558 = T18 8 items=["OUT01"=1, "OUT02"=2, "OUT03"=4, "OUT04"=8, "OUT05"=16, "OUT06"=32, "OUT07"=64, "OUT08"=128, "ALL OUT"=255] ("outNo")
        w559 = T18 4 items=["OUT01"=1, "OUT02"=2, "OUT03"=4, "OUT04"=8, "OUT05"=16, "OUT06"=32, "OUT07"=64, "OUT08"=128, "ALL OUT"=255] ("outNo")
        w560 = T18 2 items=["OUT01"=1, "OUT02"=2, "OUT03"=4, "OUT04"=8, "OUT05"=16, "OUT06"=32, "OUT07"=64, "OUT08"=128, "ALL OUT"=255] ("outNo")
        w561 = T18 1 items=["OUT01"=1, "OUT02"=2, "OUT03"=4, "OUT04"=8, "OUT05"=16, "OUT06"=32, "OUT07"=64, "OUT08"=128, "ALL OUT"=255] ("outNo")
        w562 = T18 0 items=["OUT01"=1, "OUT02"=2, "OUT03"=4, "OUT04"=8, "OUT05"=16, "OUT06"=32, "OUT07"=64, "OUT08"=128, "ALL OUT"=255] ("outNo")
        n365 = local read "select_out_command"() -> (w571:T1)
        n366 = local read "Device ID"() -> (w572:i32)
        n367 = Unbundle By Name(w571) -> ("out1"=w570:bool, "out2"=w569:bool, "out3"=w568:bool, "out4"=w567:bool, "out5"=w566:bool, "out6"=w565:bool, "out7"=w564:bool, "out8"=w563:bool)
        n368 = Select(t=w561, s=w570, f=w562) -> (s? t:f=w553:T18)
        n369 = Select(t=w560, s=w569, f=w562) -> (s? t:f=w552:T18)
        n370 = Select(t=w559, s=w568, f=w562) -> (s? t:f=w551:T18)
        n371 = Select(t=w558, s=w567, f=w562) -> (s? t:f=w550:T18)
        n372 = Select(t=w557, s=w566, f=w562) -> (s? t:f=w549:T18)
        n373 = Select(t=w556, s=w565, f=w562) -> (s? t:f=w548:T18)
        n374 = Select(t=w555, s=w564, f=w562) -> (s? t:f=w547:T18)
        n375 = Select(t=w554, s=w563, f=w562) -> (s? t:f=w546:T18)
        n376 = Compound Arithmetic op=OR(w553, w552, w551, w550, w549, w548, w547, w546) -> (w545:T18)
        n377 = case shown="\"timing_multi\"" w540 {
          tunnel: w573 -> [w581 w586 w591 w595]
          tunnel: [w581 w582 w590 w594] -> w543
          tunnel: w572 -> [_ w585 w589 w592]
          tunnel: w545 -> [_ w584 w587 w593]
          frame Default {
          }
          frame "auto_zero_multi" {
            n378 = local read "on_off"() -> (w583:bool)
            n379 = call "CL3IF_AutoZeroMulti.vi"("outNo"=w584, "error in"=w586, "onOff"=w583, "deviceId"=w585) -> ("error out"=w582:errorcluster)  [unwired: 7 in]
          }
          frame "timing_multi" {
            n380 = local read "on_off"() -> (w588:bool)
            n381 = call "CL3IF_TimingMulti.vi"("outNo"=w587, "error in"=w591, "onOff"=w588, "deviceId"=w589) -> ("error out"=w590:errorcluster)  [unwired: 7 in]
          }
          frame "reset_multi" {
            n382 = call "CL3IF_ResetMulti.vi"("outNo"=w593, "error in"=w595, "deviceId"=w592) -> ("error out"=w594:errorcluster)  [unwired: 8 in]
          }
        }
        n383 = call "set_result.vi"("error in"=w543) -> ("string"=w541:string, "font color"=w542:u32)  [unwired: 9 in]
        n384 = local write "Result_4"(w541) -> ()
        n385 = property on="Result_4" class="Str"("Text.TextColor"=w542) -> ()  [unwired: 2 in, 2 out]
      }
      frame "send_command_group" {
        w605 = T19 2 items=["GROUP1"=1, "GROUP2"=2] ("group")
        w606 = T19 1 items=["GROUP1"=1, "GROUP2"=2] ("group")
        w607 = T19 0 items=["GROUP1"=1, "GROUP2"=2] ("group")
        n386 = local read "select_group"() -> (w610:T2)
        n387 = local read "Device ID"() -> (w611:i32)
        n388 = Unbundle By Name(w610) -> ("group1"=w609:bool, "group2"=w608:bool)
        n389 = Select(t=w606, s=w609, f=w607) -> (s? t:f=w604:T19)
        n390 = Select(t=w605, s=w608, f=w607) -> (s? t:f=w603:T19)
        n391 = Compound Arithmetic op=OR(w604, w603) -> (w602:T19)
        n392 = case shown="\"auto_zero_group\"" w597 {
          tunnel: w612 -> [w620 w625 w630 w633]
          tunnel: [w620 w624 w629 w632] -> w600
          tunnel: w611 -> [_ w623 w627 w631]
          tunnel: w602 -> [_ w622 w626 w634]
          frame Default {
          }
          frame "auto_zero_group" {
            n393 = local read "on_off_group"() -> (w621:bool)
            n394 = call "CL3IF_AutoZeroGroup.vi"("group"=w622, "error in"=w625, "onOff"=w621, "deviceId"=w623) -> ("error out"=w624:errorcluster)  [unwired: 7 in]
          }
          frame "timing_group" {
            n395 = local read "on_off_group"() -> (w628:bool)
            n396 = call "CL3IF_TimingGroup.vi"("group"=w626, "error in"=w630, "onOff"=w628, "deviceId"=w627) -> ("error out"=w629:errorcluster)  [unwired: 7 in]
          }
          frame "reset_group" {
            n397 = call "CL3IF_ResetGroup.vi"("group"=w634, "error in"=w633, "deviceId"=w631) -> ("error out"=w632:errorcluster)  [unwired: 8 in]
          }
        }
        n398 = call "set_result.vi"("error in"=w600) -> ("string"=w598:string, "font color"=w599:u32)  [unwired: 9 in]
        n399 = local write "Result_4"(w598) -> ()
        n400 = property on="Result_4" class="Str"("Text.TextColor"=w599) -> ()  [unwired: 2 in, 2 out]
      }
      frame "send_command_program" {
        n401 = local read "Device ID"() -> (w645:i32)
        n402 = case shown="\"switch_program\"" w640 {
          tunnel: w646 -> [w652 w660 w673]
          tunnel: [w652 w656 w672] -> w643
          tunnel: w645 -> [_ w659 w671]
          tunnel: w638 -> [w651 w653 w669]
          tunnel: [w651 w655 w669] -> w637
          tunnel: w636 -> [_ w654 _]
          frame Default {
          }
          frame "switch_program" {
            n403 = local read "switch_program_no"() -> (w658:u8)
            n404 = call "CL3IF_SwitchProgram.vi"("error in"=w660, "programNo"=w658, "deviceId"=w659) -> ("error out"=w657:errorcluster)  [unwired: 8 in]
            n405 = case shown="True" w654 {
              tunnel: w657 -> [w662 w667]
              tunnel: [w662 w666] -> w656
              tunnel: [w661 w665] -> w655
              tunnel: w653 -> [w661 _]
              frame False {
              }
              frame True {
                n406 = local read "Device ID"() -> (w668:i32)
                n407 = local write "data num"(u16 0 ("data num")) -> ()
                n408 = call "CL3IF_GetTrendIndex.vi"("error in"=w667, "deviceId"=w668) -> ("error out"=w666:errorcluster, "index"=w665:u32)  [unwired: 8 in]
                n409 = local write "Trend Graph"(T8 [{array[10000 elements]}, {array[10000 elements]}, {array[10000 elements]}, {array[10000 elements]}, {array[10000 elements]}, {array[10000 elements]}, {array[10000 elements]}, {array[10000 elements]}]) -> ()
              }
            }
          }
          frame "get_program_no" {
            n410 = call "CL3IF_GetProgramNo.vi"("error in"=w673, "deviceId"=w671) -> ("error out"=w672:errorcluster, "programNo"=w670:u8)  [unwired: 8 in]
            n411 = local write "program_no"(w670) -> ()
          }
        }
        n412 = call "set_result.vi"("error in"=w643) -> ("string"=w641:string, "font color"=w642:u32)  [unwired: 9 in]
        n413 = local write "Result_5"(w641) -> ()
        n414 = property on="Result_5" class="Str"("Text.TextColor"=w642) -> ()  [unwired: 2 in, 2 out]
      }
      frame "send_command_pulse" {
        n415 = local read "Device ID"() -> (w680:i32)
        n416 = case shown="\"get_pulse_count\"" w675 {
          tunnel: w681 -> [w689 w693 w699]
          tunnel: [w689 w692 w698] -> w678
          tunnel: w680 -> [_ w691 w697]
          frame Default {
          }
          frame "get_pulse_count" {
            n417 = call "CL3IF_GetPulseCount.vi"("error in"=w693, "deviceId"=w691) -> ("error out"=w692:errorcluster, "pulseCount"=w690:i32)  [unwired: 8 in]
            n418 = local write "pulse_count"(w690) -> ()
          }
          frame "reset_pulse_count" {
            n419 = local write "data num"(u16 0 ("data num")) -> ()
            n420 = local write "pulase_reset"(TRUE) -> ()
            n421 = call "CL3IF_ResetPulseCount.vi"("error in"=w699, "deviceId"=w697) -> ("error out"=w698:errorcluster)  [unwired: 9 in]
            n422 = local write "Trend Graph"(T8 [{array[10000 elements]}, {array[10000 elements]}, {array[10000 elements]}, {array[10000 elements]}, {array[10000 elements]}, {array[10000 elements]}, {array[10000 elements]}, {array[10000 elements]}]) -> ()
          }
        }
        n423 = call "set_result.vi"("error in"=w678) -> ("string"=w676:string, "font color"=w677:u32)  [unwired: 9 in]
        n424 = local write "Result_6"(w676) -> ()
        n425 = property on="Result_6" class="Str"("Text.TextColor"=w677) -> ()  [unwired: 2 in, 2 out]
      }
      frame "send_command_ctrl" {
        n426 = local read "Device ID"() -> (w706:i32)
        n427 = case shown="\"meas_ctrl_off\"" w701 {
          tunnel: w707 -> [w715 w719 w723 w727 w731]
          tunnel: [w715 w718 w722 w726 w730] -> w704
          tunnel: w706 -> [_ w717 w721 w725 w729]
          frame Default {
          }
          frame "meas_ctrl_on" {
            n428 = call "CL3IF_MeasurementControl.vi"("error in"=w719, "onOff"=TRUE, "deviceId"=w717) -> ("error out"=w718:errorcluster)  [unwired: 8 in]
          }
          frame "meas_ctrl_off" {
            n429 = call "CL3IF_MeasurementControl.vi"("error in"=w723, "onOff"=FALSE, "deviceId"=w721) -> ("error out"=w722:errorcluster)  [unwired: 8 in]
          }
          frame "light_ctrl_on" {
            n430 = call "CL3IF_LightControl.vi"("error in"=w727, "onOff"=TRUE, "deviceId"=w725) -> ("error out"=w726:errorcluster)  [unwired: 8 in]
          }
          frame "light_ctrl_off" {
            n431 = call "CL3IF_LightControl.vi"("error in"=w731, "onOff"=FALSE, "deviceId"=w729) -> ("error out"=w730:errorcluster)  [unwired: 8 in]
          }
        }
        n432 = call "set_result.vi"("error in"=w704) -> ("string"=w702:string, "font color"=w703:u32)  [unwired: 9 in]
        n433 = local write "Result_7"(w702) -> ()
        n434 = property on="Result_7" class="Str"("Text.TextColor"=w703) -> ()  [unwired: 2 in, 2 out]
      }
      frame "send_command_clear_storage" {
        n435 = local read "Device ID"() -> (w738:i32)
        n436 = case shown="\"clear_storage_data\"" w735 {
          tunnel: w739 -> [w747 w750]
          tunnel: [w747 w749] -> w736
          tunnel: w738 -> [_ w748]
          frame Default {
          }
          frame "clear_storage_data" {
            n437 = call "CL3IF_ClearStorageData.vi"("error in"=w750, "deviceId"=w748) -> ("error out"=w749:errorcluster)  [unwired: 9 in]
          }
        }
        n438 = call "set_result.vi"("error in"=w736) -> ("string"=w733:string, "font color"=w734:u32)  [unwired: 9 in]
        n439 = local write "Result_3"(w733) -> ()
        n440 = property on="Result_3" class="Str"("Text.TextColor"=w734) -> ()  [unwired: 2 in, 2 out]
      }
      frame "save_csv_file" {
        n441 = local read "path"() -> (w753:path)
        n442 = call <vilib>:"Check if File or Folder Exists.vi"("error in (no error)"=w757, "path"=w753) -> ("error out"=w756:errorcluster, "file or folder exists?"=w755:bool)  [unwired: 7 in, 1 out]
        n443 = Empty String/Path?(string/path=w753) -> (empty?=w752:bool)
        n444 = Not(x=w752) -> (.not. x?=w751:bool)
        n445 = And(x=w755, y=w751) -> (x .and. y?=w754:bool)
        n446 = case shown="True" w754 {
          tunnel: w756 -> [w769 w779]
          tunnel: [w769 w778] -> w758
          frame False {
            n447 = One Button Dialog(message="File save folder not found" ("メッセージ")) -> ()  [unwired: 1 in, 1 out]
          }
          frame True {
            n448 = local read "select_out_last"() -> (w771:T1)
            n449 = Cluster To Array(cluster=w771) -> (array=w775:bool[])
            n450 = for {
              tunnel: w775 -> [w791] mode=indexing
              shift-right: [w790] -> w773
              shift-left: u8 0 -> [w789]
              n451 = Increment(x=w789) -> (x+1=w788:u8)
              n452 = Select(t=w788, s=w791, f=w789) -> (s? t:f=w790:u8)
            }
            n453 = case shown="8" w773 {
              tunnel: [w780 w781 w782 w783 w784 w785 w786 w787] -> w772
              frame 0, 1, Default {
                n454 = property on="log1" class="WFChart (strict)"() -> ("History Data"=w780:dbl[][])  [unwired: 2 in, 2 out]
              }
              frame 2 {
                n455 = property on="log2" class="WFChart (strict)"() -> ("History Data"=w781:dbl[][])  [unwired: 2 in, 2 out]
              }
              frame 3 {
                n456 = property on="log3" class="WFChart (strict)"() -> ("History Data"=w782:dbl[][])  [unwired: 2 in, 2 out]
              }
              frame 4 {
                n457 = property on="log4" class="WFChart (strict)"() -> ("History Data"=w783:dbl[][])  [unwired: 2 in, 2 out]
              }
              frame 5 {
                n458 = property on="log5" class="WFChart (strict)"() -> ("History Data"=w784:dbl[][])  [unwired: 2 in, 2 out]
              }
              frame 6 {
                n459 = property on="log6" class="WFChart (strict)"() -> ("History Data"=w785:dbl[][])  [unwired: 2 in, 2 out]
              }
              frame 7 {
                n460 = property on="log7" class="WFChart (strict)"() -> ("History Data"=w786:dbl[][])  [unwired: 2 in, 2 out]
              }
              frame 8 {
                n461 = property on="log8" class="WFChart (strict)"() -> ("History Data"=w787:dbl[][])  [unwired: 2 in, 2 out]
              }
            }
            n462 = local read "path"() -> (w776:path)
            n463 = property on="Trend Graph" class="XYGraph (strict)"() -> ("XScale.NameLbl.Text"=w777:string)  [unwired: 2 in, 2 out]
            n464 = call "save_csv_file.vi"("Data"=w772, "error in"=w779, "select_out_graph"=w771, "Graph"=w777, "Path"=w776) -> ("error out"=w778:errorcluster)  [unwired: 6 in]
          }
        }
      }
      frame "error" {
        n465 = call <vilib>:"Clear Errors.vi"("error in (no error)"=w801) -> ("error out"=w800:errorcluster)  [unwired: 5 in, 1 out]
      }
      frame "end" {
        w808 = T5."Enabled"
        w811 = FALSE
        w813 = T5."Disabled and Grayed Out"
        w812 = T5."Enabled"
        w817 = u32 0 ("Index")
        w814 = FALSE
        n466 = local read "Device ID"() -> (w805:i32)
        n467 = property on="No Wave" class="Str"("Visible"=FALSE) -> ()  [unwired: 2 in, 2 out]
        n468 = property on="mask_left_1" class="Bool (strict)"("Visible"=w811) -> ()  [unwired: 2 in, 2 out]
        n469 = property on="mask_right" class="Bool (strict)"("Visible"=w811) -> ()  [unwired: 2 in, 2 out]
        n470 = property on="mask_left_2" class="Bool (strict)"("Visible"=w811) -> ()  [unwired: 2 in, 2 out]
        n471 = call "CL3IF_StopStorage.vi"("error in"=w810, "deviceId"=w805) -> ("error out"=w809:errorcluster)  [unwired: 9 in]
        n472 = call <vilib>:"Clear Errors.vi"("error in (no error)"=w809) -> ("error out"=w806:errorcluster)  [unwired: 5 in, 1 out]
        n473 = property on="open" class="Bool"("DisabledEnum"=w812) -> ()  [unwired: 2 in, 2 out]
        n474 = property on="Comm Interface" class="Enum (strict)"("DisabledEnum"=w812) -> ()  [unwired: 2 in, 2 out]
        n475 = property on="Device ID" class="DigNum (strict)"("DisabledEnum"=w812) -> ()  [unwired: 2 in, 2 out]
        n476 = property on="IP Address" class="Arr (strict)"("DisabledEnum"=w812) -> ()  [unwired: 2 in, 2 out]
        n477 = property on="Port" class="DigNum (strict)"("DisabledEnum"=w812) -> ()  [unwired: 2 in, 2 out]
        n478 = property on="timeout" class="DigNum (strict)"("DisabledEnum"=w812) -> ()  [unwired: 2 in, 2 out]
        n479 = call "Close.vi"("error in (no error)"=w806, "deviceId"=w805) -> ("error out"=w804:errorcluster)  [unwired: 9 in]
        n480 = call <vilib>:"Clear Errors.vi"("error in (no error)"=w804) -> ()  [unwired: 5 in, 2 out]
        n481 = property on="get_trend_start" class="Bool"("DisabledEnum"=w808) -> ()  [unwired: 2 in, 2 out]
        n482 = property on="start_storage" class="Bool"("DisabledEnum"=w808) -> ()  [unwired: 2 in, 2 out]
        n483 = property on="get_storage_data" class="Bool"("DisabledEnum"=w808) -> ()  [unwired: 2 in, 2 out]
        n484 = property on="clear_storage_data" class="Bool"("DisabledEnum"=w808) -> ()  [unwired: 2 in, 2 out]
        n485 = property on="get_light_start" class="Bool"("DisabledEnum"=w808) -> ()  [unwired: 2 in, 2 out]
        n486 = property on="select_graph" class="Enum (strict)"("DisabledEnum"=w808) -> ()  [unwired: 2 in, 2 out]
        n487 = property on="select_out_graph" class="Clust (strict)"("DisabledEnum"=w808) -> ()  [unwired: 2 in, 2 out]
        n488 = property on="close" class="Bool"("DisabledEnum"=w813) -> ()  [unwired: 2 in, 2 out]
        n489 = property on="stop_storage" class="Bool"("DisabledEnum"=w813) -> ()  [unwired: 2 in, 2 out]
        n490 = property on="get_trend_stop" class="Bool"("DisabledEnum"=w813) -> ()  [unwired: 2 in, 2 out]
        n491 = property on="get_light_stop" class="Bool"("DisabledEnum"=w813) -> ()  [unwired: 2 in, 2 out]
      }
    }
  }
